vi "Filter Wheel GUI.vi"(9 "Standalone":bool=TRUE, 10 "Init Data":variant, 11 "Filter Wheel name":string="RIMAS") -> ()   [LabVIEW 2024]
uses:
  Filter Wheel Arduino Control/Filter Wheel Arduino Command cluster.ctl
  typedefs/CC enum Operation Mode.ctl
  Filter Wheel Arduino Control/Filter Wheel Arduino Homing cluster.ctl
  Filter Wheel Object/Filter Wheel.lvclass
  Filter Wheel configuration.ctl
  Filter Wheel Object/Filter Wheel Details.ctl
  Subsystems/SS typedef cluster Instrument Command Queue Data.ctl
  Subsystems/SS cluster Data Queue type.ctl
  FW cmd Q Move Parameters.ctl
  <vilib>/Utility/miscctls.llb/LVRowAndColumnTypeDef.ctl
  FW cluster Status.ctl
  FW enum status.ctl
  Filter Wheel Object/Filter Wheel.lvclass/Filter Wheel.ctl
  hk-channel-class/hk-channel-class/HK Item/HK Channel Units and Setup.ctl
  hk-channel-class/hk-channel-class/HK Item/HK Channel enum Data Type.ctl
  hk-channel-class/hk-channel-class/HK Item/HK Item.lvclass
  hk-channel-class/hk-channel-class/HK Item/HK Channel cluster Telemetry Data.ctl
  FW cmd Q Move Position Parameters.ctl
  typedefs/CC cluster Alarm Data.ctl
  Filter Wheel Arduino Control/FW Arduino Control.lvclass
  Filter Wheel Simulator/Filter Wheel Simulator.lvclass
  C:/Development/rimas/RIMAS/Filter Wheel/Filter Wheel Object/Filter Wheel.lvclass
  Filter Wheel Simulator/Filter Wheel Simulator.lvclass/Filter Wheel Simulator.ctl
panel:
  out "Messages":string
  in  "Mode":T1
  in  "Tab Control":T2(tab)
  out "Wheel Name":string
  out "Moving Message":string="Filter Wheel Moving...."
  in  "Error":bool
  out "Homed":bool[](array[boolean])
  in  "Wheel To Home":u16(ring) items=["FW YJ", "FW HK", "Aux", "Slit"]
  in  "STOP":bool
  out "Connected":bool
  in  "Filter Wheel Displays":T3 {"Gauge 0" scale=0.0..5.0; "Gauge 4" scale=0.0..5.0; "Gauge 3" scale=0.0..6.0; "Gauge 2" scale=0.0..5.0; "Gauge 5" scale=0.0..32768.0; "Gauge 8" scale=0.0..32768.0; "Gauge 6" scale=0.0..32768.0; "Gauge 7" scale=0.0..32768.0}
  in  "Home":bool
  out "Repeats":i32
  in  "Wheel ID":i32
  in  "Repeat Home":bool
  in  "Alarms?":bool=TRUE
  in  "Default Speed":u16=200 min=20 max=4000 step=10
  in  "Homing":T4[](array[typedef])
  in  "Sim Velocity (steps/sec)":i32
  in  "Connect":bool
  in  "Serial Port":refnum<visa-resource-name>="COM11"
  in  "Simulate":bool
  in  "Close":bool
  in  "Filter Wheel":u16(ring)
  in  "Slit Wheel Location":u16(ring)
  in  "Save Slit Wheel Pos":bool
  in  "Open Arduino Log":bool
  out "Moving":bool[](array[boolean])
  out "Last Move Positions":u32[](array[numeric])
  out "On the notch":bool[](array[boolean])
  in  "Filter Wheel Settings":T5={"Direction"=TRUE, "NUMBER OF  STEPS"=2900, "SPEED STEPS/SEC"=200, "ACC/DECEL STEPS/SEC^2"=400, "Move mode"=0, "EN/DIS?"=TRUE, "delay before \nread (ms)"=750, "Timeout before \nstop (ms)"=13000} {"Move mode" items=["Relative steps ##", "Search switch"]; "ACC/DECEL STEPS/SEC^2" max=4000; "SPEED STEPS/SEC" min=20 max=4000 step=10}
  in  "Command Preview":string
  out "Response":string
  in  "Send Command":bool
  in  "Read":bool
  in  "Restore Defaults":bool
  in  "Remove Pos":bool
  in  "Add Pos":bool
  in  "Save Button":bool
  in  "Remove Fw":bool
  in  "Add Fw":bool
  in  "Wheels":i32(listbox)
  in  "Positions":i32(listbox)
  # "Click for info"
  # "Home button will repeatedly home the wheel until it is pressed again. Repeats show number of homes done so far."
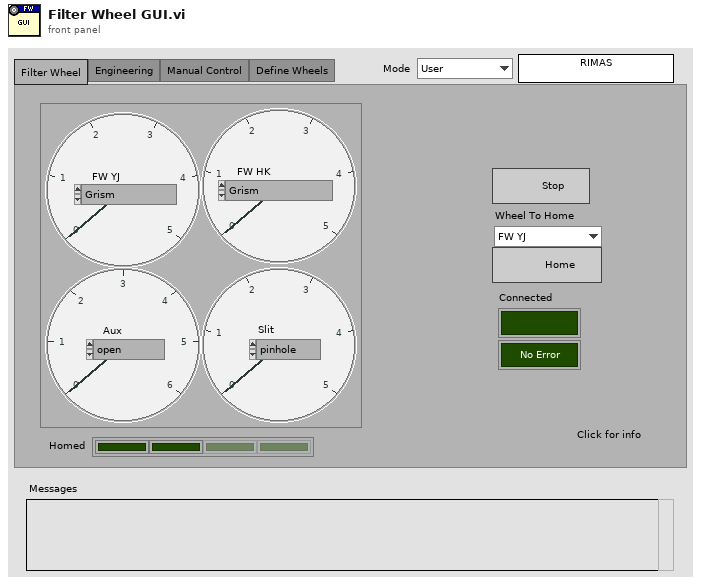
[diagram p1: front panel]
types:
  T1 = typedef "CC enum Operation Mode.ctl" = enum16{"User", "Engineering"}
  T2 = enum32{"Filter Wheel", "Engineering", "Manual Control", "Define Wheels"}
  T3 = cluster{"Gauge 0":i32, "Gauge 2":i32, "Gauge 3":i32, "Gauge 4":i32, "Gauge 5":i32, "Gauge 6":i32, "Gauge 7":i32, "Gauge 8":i32, "Position 0":i32, "Position 1":i32, "Position 2":i32, "Position 3":i32}
  T4 = typedef "Filter Wheel Arduino Homing cluster.ctl" = cluster{"Direction":bool, "Speed":i32, "Accel":i32, "Error Cnts":i32, "Homing Delta":i32}
  T5 = typedef "Filter Wheel Arduino Command cluster.ctl" = cluster{"Direction":bool, "NUMBER OF  STEPS":u32, "SPEED STEPS/SEC":u16, "ACC/DECEL STEPS/SEC^2":u16, "Move mode":u16, "EN/DIS?":bool, "delay before \nread (ms)":u32, "Timeout before \nstop (ms)":u32}
  T6 = typedef "SS typedef cluster Instrument Command Queue Data.ctl" = cluster{"Cmd":string, "Parameters":variant}
  T7 = typedef "Filter Wheel.lvclass/Filter Wheel configuration.ctl" = cluster{"Num Wheels":i32, "Filters":T8[], "Invalid Combinations":i32[][], "Addr":refnum<visa-resource-name>, "Name":string, "Simulate":bool, "Default Speed":u16, "Homing":T4[]}
  T8 = typedef "Filter Wheel.lvclass/Filter Wheel Details.ctl" = cluster{"Names":string[], "Relative Position":i32[], "Wheel Name":string, "Size":i32}
  T9 = typedef "FW cmd Q Move Parameters.ctl" = cluster{"Wheel ID":i32, "Position":i32}
  T10 = typedef "LVRowAndColumnTypeDef.ctl" = cluster{"Row":i32, "Column":i32}
  T11 = typedef "FW cluster Status.ctl" = cluster{"State":T12, "Positions":i32[], "Names":string[], "Notch":bool[], "Moving":bool[]}
  T12 = typedef "FW enum status.ctl" = enum16{"Initializing", "Moving", "Move Complete", "Error"}
  T13 = cluster{"state":refnum<user-event>, "Filter Wheel ref":refnum<class "Filter Wheel.lvclass">, "Filter Wheel Info":T7, "FW names":string[], "Pos Names":cluster{"Table":string[][]}[], "cmd q":refnum<queue>, "Cmd":T6, "Data Q":refnum<queue>, "Move":T9, "error":errorcluster, "next poll":timestamp, "FW refs":refnum<vi>[], "Wheel":i32, "Coords":T10, "fw name":string, "Simulate":bool, "ch names":string[][], "FW Status":T11, "Error State":string, "Name":string, "Period":dbl, "Home Repeats":i32}
  T14 = typedef "HK Item.lvclass/HK Channel Units and Setup.ctl" = cluster{"Unit Type":string, "Units":string, "Configuration":string, "Digits":i32, "Data Type":T15, "Exponential?":bool, "Source":string}
  T15 = typedef "HK Item.lvclass/HK Channel enum Data Type.ctl" = enum16{"Floating Point", "Integer", "Enum", "String", "Waveform", "File"}
  T16 = typedef "SS cluster Data Queue type.ctl" = cluster{"Source":string, "Type":string, "Data":variant}
  T17 = typedef "HK Item.lvclass/HK Channel cluster Telemetry Data.ctl" = cluster{"Ch Names":string[], "Ch Values":dbl[], "Timestamp":timestamp, "Data Type":T15}
  T18 = typedef "FW cmd Q Move Position Parameters.ctl" = cluster{"Position Names":string[]}
  T19 = enum32{"Page Enabled", "Page Disabled", "Page Disabled & Grayed"}
  T20 = typedef "CC cluster Alarm Data.ctl" = cluster{"Measured Value":dbl, "Alarm Low":dbl, "Alarm High":dbl, "Message":string, "Source":string}
  T21 = enum8{"Enabled", "Disabled", "Disabled and Grayed Out"}
  T22 = typedef "LVPoint32TypeDef.ctl" = cluster{"Horizontal":i32, "Vertical":i32}
  T23 = cluster{"Gauge 0":bool, "Gauge 2":bool, "Gauge 3":bool, "Gauge 4":bool, "Gauge 5":bool, "Gauge 6":bool, "Gauge 7":bool, "Gauge 8":bool, "Position 0":bool, "Position 1":bool, "Position 2":bool, "Position 3":bool}
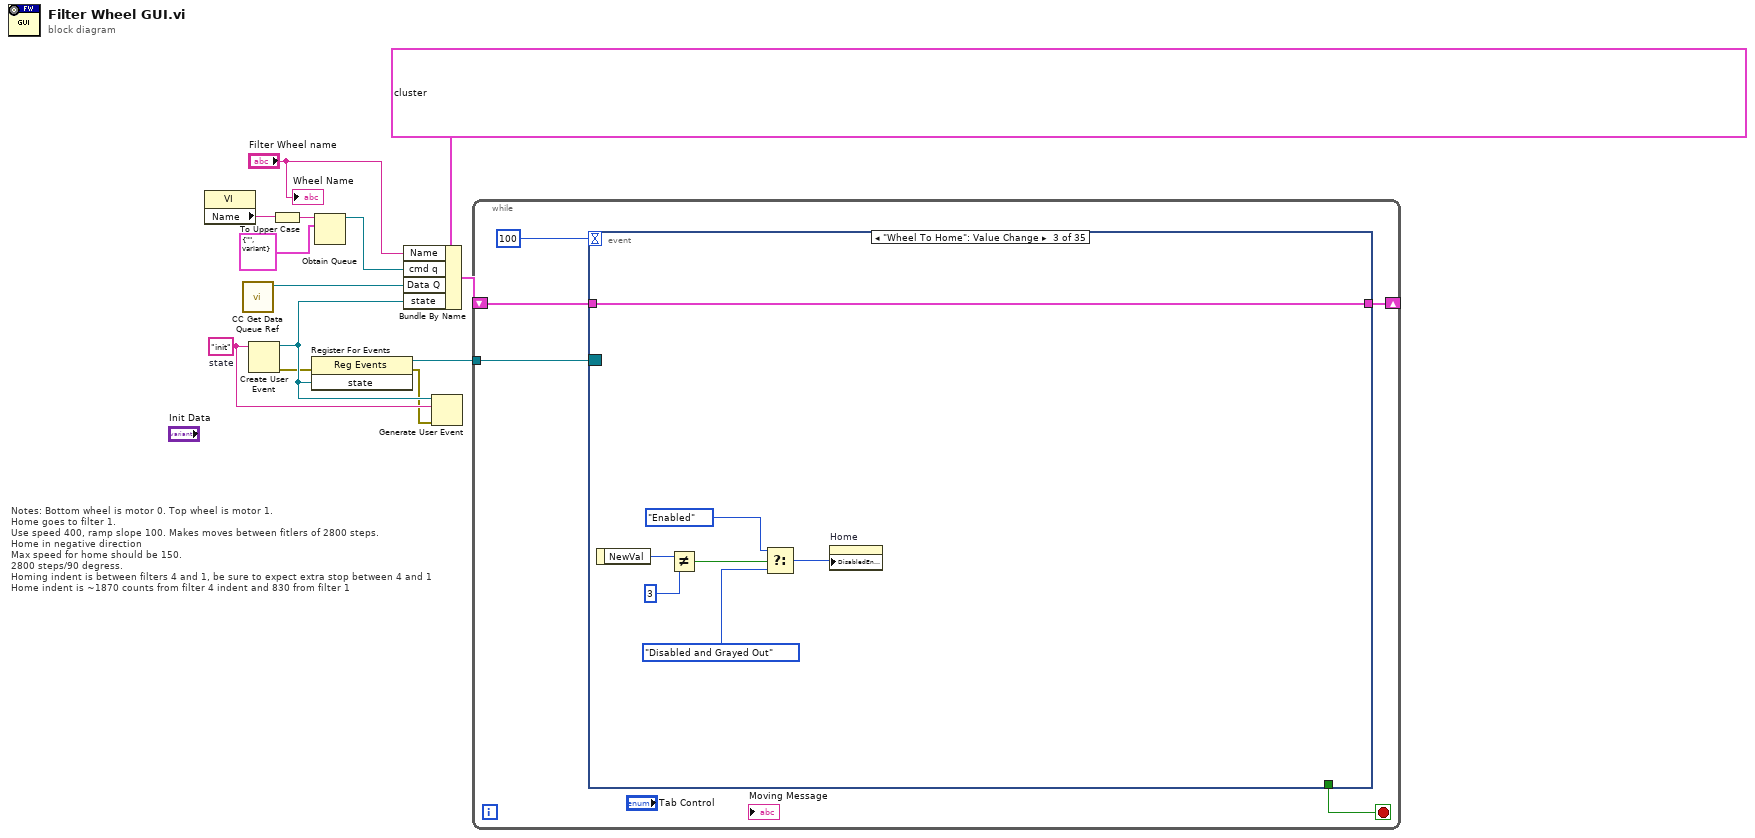
[diagram p0: block diagram]
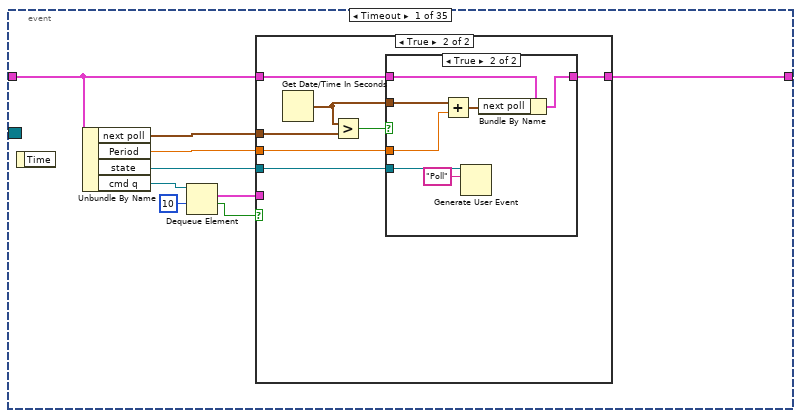
[diagram p2: hidden frame]
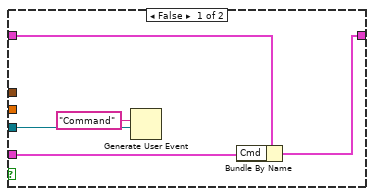
[diagram p3: hidden frame]
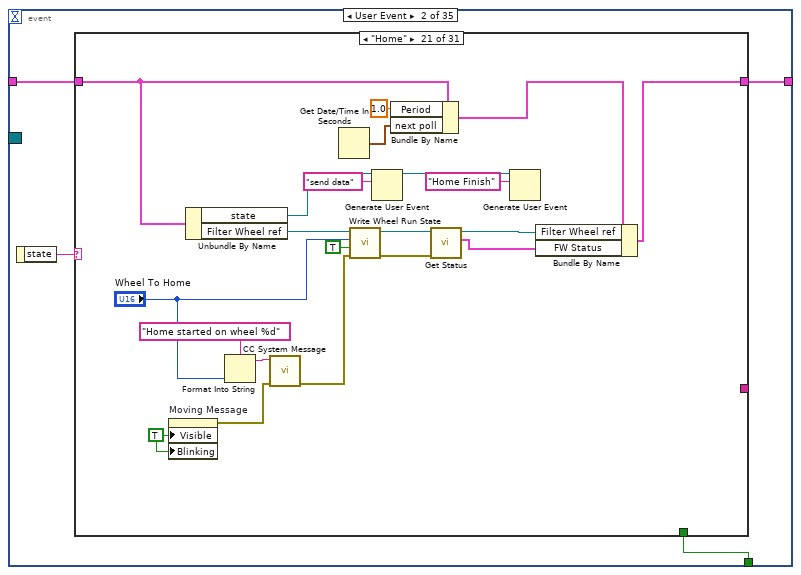
[diagram p5: hidden frame]
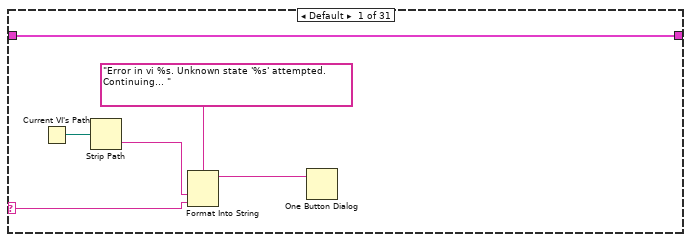
[diagram p6: hidden frame]
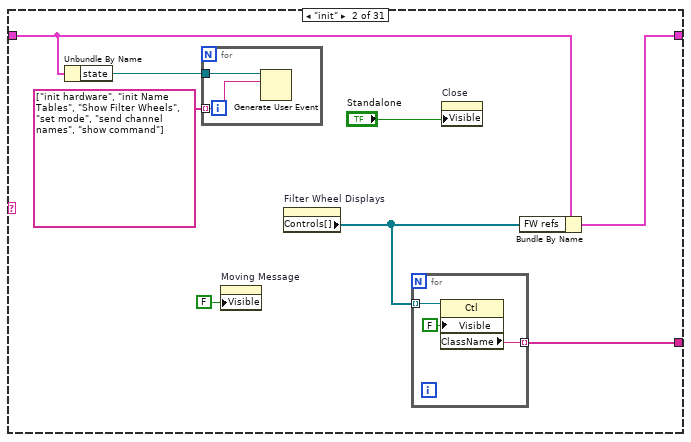
[diagram p7: hidden frame]
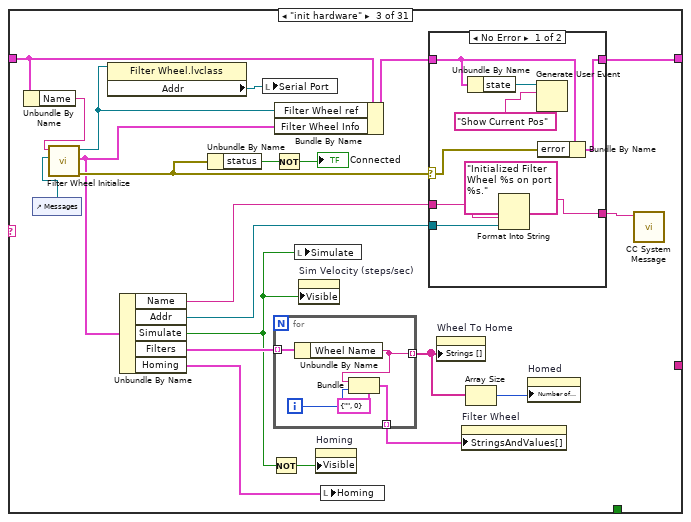
[diagram p8: hidden frame]
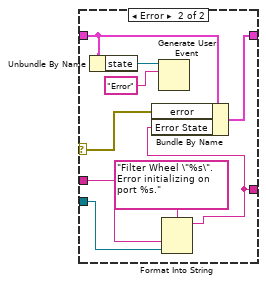
[diagram p9: hidden frame]
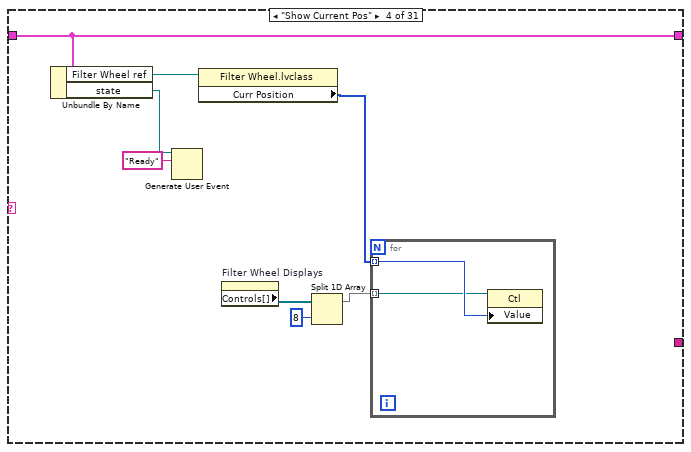
[diagram p10: hidden frame]
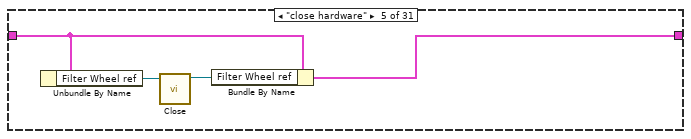
[diagram p11: hidden frame]
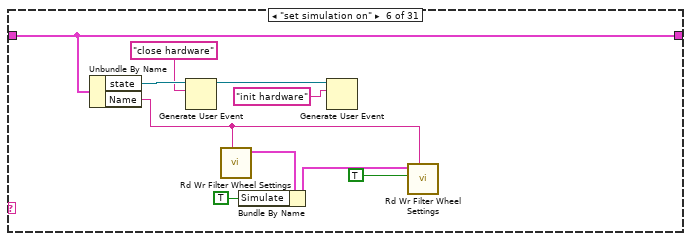
[diagram p12: hidden frame]
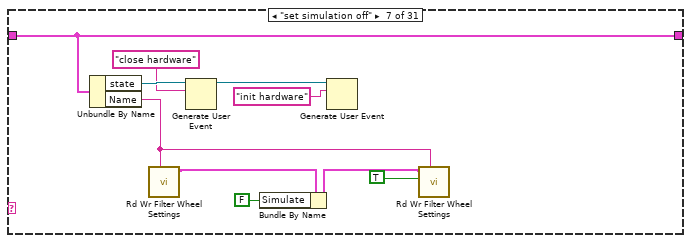
[diagram p13: hidden frame]
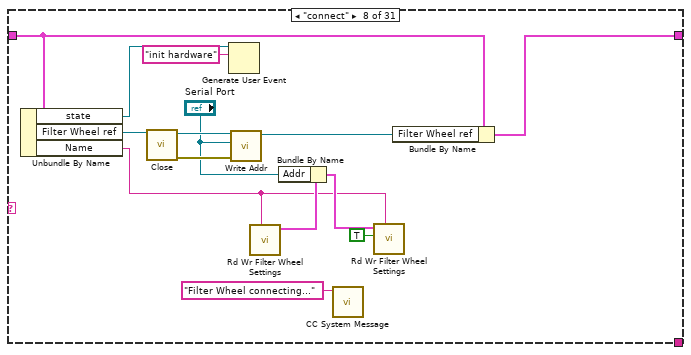
[diagram p14: hidden frame]
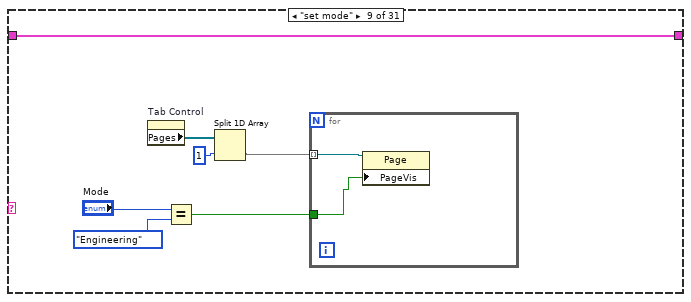
[diagram p15: hidden frame]
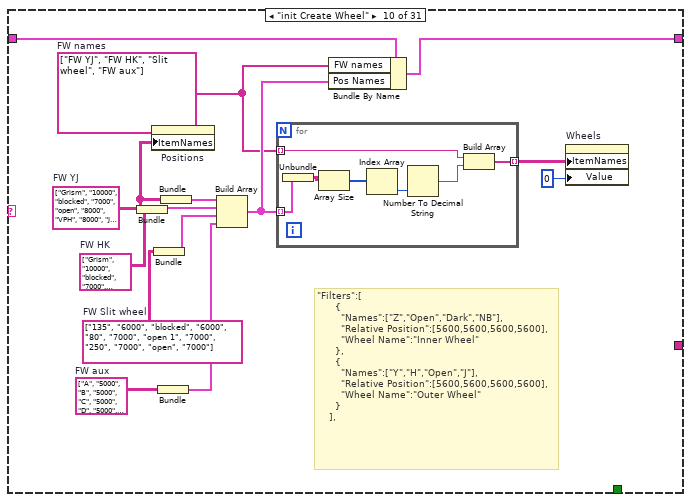
[diagram p16: hidden frame]
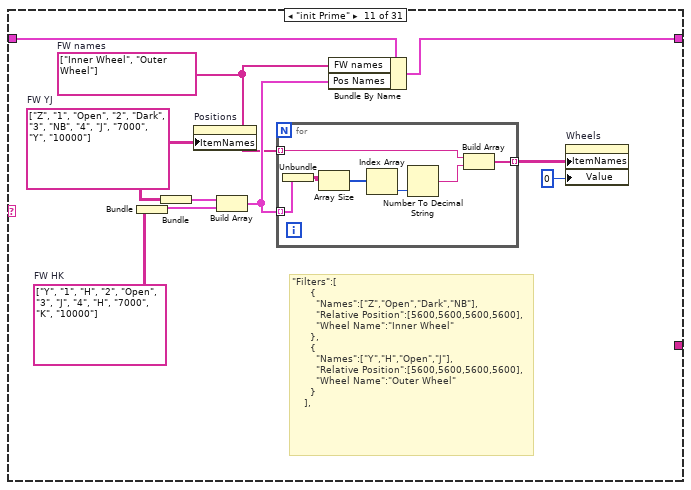
[diagram p17: hidden frame]
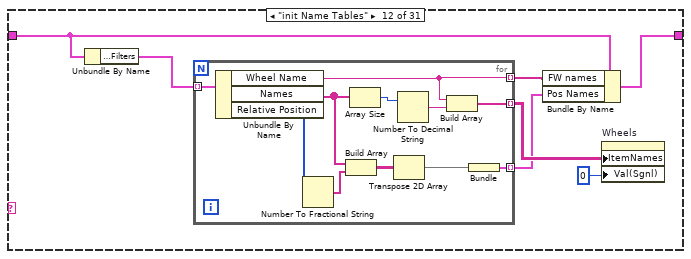
[diagram p18: hidden frame]
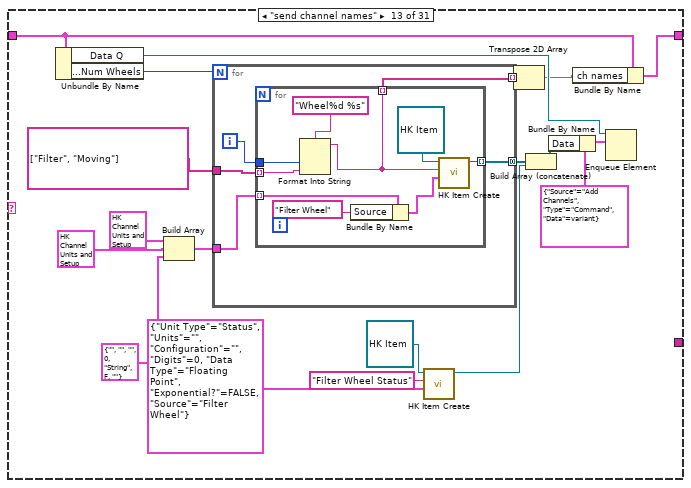
[diagram p19: hidden frame]
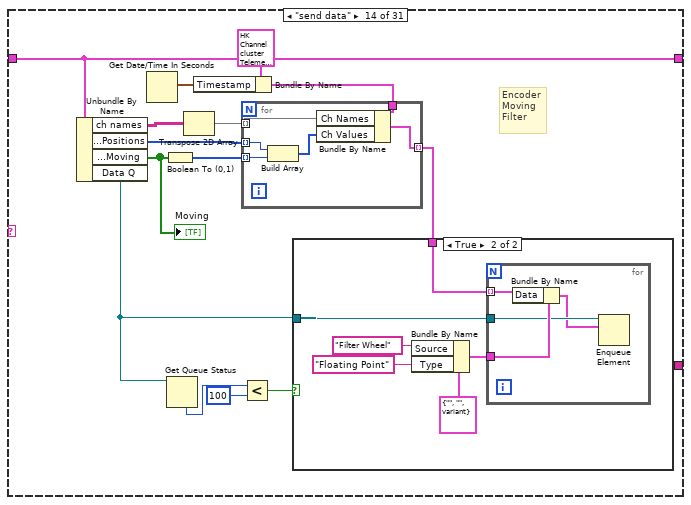
[diagram p20: hidden frame]
diagram:
  w9 = "init"  # state
  # "Notes: Bottom wheel is motor 0. Top wheel is motor 1.\nHome goes to filter 1. \nUse speed 400, ramp slope 100. Makes moves between fitlers of 2800 steps.\nHome in negative direction\nMax speed for home should be 150.\n2800 steps/90 degress.\nHoming indent is between filters 4 and 1, be sure to expect extra stop between 4 and 1\nHome indent is ~1870 counts from filter 4 indent and 830 from filter 1"
  n1 = property class="VI"() -> ("Name"=w5:string)  [unwired: 2 in, 2 out]
  n2 = call "CC Get Data Queue Ref.vi"() -> ("Data Q"=w6:refnum<queue>)  [unwired: 10 in, 1 out]
  n3 = Create User Event(user event datatype=w9) -> (user event=w11:refnum<user-event>, error out=w7:errorcluster)  [unwired: 1 in]
  n4 = To Upper Case(1:w5) -> (0:w4:string)
  n5 = register-events(error in=w7, w11) -> (reference out=w10:refnum<event-registration>, error out=w8:errorcluster)  [unwired: 1 in]
  n6 = Obtain Queue(name (unnamed)=w4, element data type=T6 {"Cmd"="", "Parameters"=variant}) -> (queue out=w2:refnum<queue>)  [unwired: 3 in, 2 out]
  n7 = Bundle By Name(cluster=T13 {"state"=refnum, "Filter Wheel ref"=refnum, "Filter Wheel Info"={"Num Wheels"=0, "Filters"=[], "Invalid Combinations"=[], "Addr"="", "Name"="", "Simulate"=FALSE, "Default Speed"=1000, "Homing"=[]}, "FW names"=["FW YJ", "FW HK", "Slit wheel", "FW aux"], "Pos Names"=[], "cmd q"=refnum, "Cmd"={"Cmd"="", "Parameters"=variant}, "Data Q"=refnum, "Move"={"Wheel ID"=0, "Position"=0}, "error"={"status"=FALSE, "code"=0, "source"=""}, "next poll"=timestamp(0 s since 1904-01-01), "FW refs"=[], "Wheel"=0, "Coords"={"Row"=0, "Column"=0}, "fw name"="", "Simulate"=TRUE, "ch names"=[], "FW Status"={"State"=enum."Move Complete", "Positions"=[], "Names"=[], "Notch"=[], "Moving"=[FALSE, FALSE]}, "Error State"="", "Name"="PRIME", "Period"=10.0, "Home Repeats"=0}, "Name"="Filter Wheel name", "cmd q"=w2, "Data Q"=w6, "state"=w11) -> (w12:T13)
  n8 = Generate User Event(user event=w11, event data cluster=w9, error in=w8) -> ()  [unwired: 1 in, 2 out]
  n9 = while {
    tunnel: w10 -> [w18]
    shift-right: [w17] -> _
    shift-left: w12 -> [w14]
    stop <- w16 stop-if-true
    n10 = event shown="[2] \"Wheel To Home\": Value Change" {
      selector: w18 -> [_ _ _ _ _ _ _ _ _ _ _ _ _ _ _ _ _ _ _ _ _ _ _ _ _ _ _ _ _ _ _ _ _ _ _]
      dyn-events: _ -> [_ _ _ _ _ _ _ _ _ _ _ _ _ _ _ _ _ _ _ _ _ _ _ _ _ _ _ _ _ _ _ _ _ _ _]
      timeout: 100 -> [_ _ _ _ _ _ _ _ _ _ _ _ _ _ _ _ _ _ _ _ _ _ _ _ _ _ _ _ _ _ _ _ _ _ _]
      tunnel: w14 -> [w22 w50 w608 w614 w618 w624 w644 w646 w655 w658 w660 w682 w689 w698 w701 w709 w710 w725 w728 w731 w734 w737 w746 w750 w757 w767 w789 w805 w827 w836 w842 w865 w878 w899 w903]
      tunnel: [w21 w49 w608 w613 w619 w625 w644 w645 w655 w658 w663 w683 w690 w698 w701 w709 w711 w725 w728 w731 w734 w737 w747 w751 w758 w768 w790 w806 w828 w837 w843 w866 w879 w899 w903] -> w17
      tunnel: [_ w48 _ _ _ _ _ _ _ _ _ _ _ _ _ _ _ _ _ _ _ _ _ _ _ _ _ _ _ _ _ _ _ _ _] -> w16
      event Timeout {
        n11 = event-data() -> ()  [unwired: 1 in, 1 out]
        n12 = Unbundle By Name(w22) -> ("next poll"=w20:timestamp, "Period"=w19:dbl, "state"=w23:refnum<user-event>, "cmd q"=w27:refnum<queue>)
        n13 = Dequeue Element(queue=w27, timeout in ms (-1)=10) -> (element=w24:T6, timed out?=w25:bool)  [unwired: 1 in, 2 out]
        n14 = case shown="True" w25 {
          tunnel: w24 -> [w29 _]
          tunnel: w23 -> [w32 w36]
          tunnel: w22 -> [w30 w37]
          tunnel: [w28 w34] -> w21
          tunnel: w20 -> [_ w39]
          tunnel: w19 -> [_ w33]
          frame False {
            n15 = Generate User Event(user event=w32, event data cluster="Command" ("event data")) -> ()  [unwired: 2 in, 2 out]
            n16 = Bundle By Name(cluster=w30, "Cmd"=w29) -> (w28:T13)
          }
          frame True {
            n17 = Get Date/Time In Seconds() -> (seconds since 1Jan1904=w35:timestamp)
            n18 = Greater?(x=w35, y=w39) -> (0:w38:bool)
            n19 = case shown="True" w38 {
              tunnel: w37 -> [w40 w47]
              tunnel: w36 -> [_ w46]
              tunnel: w35 -> [_ w45]
              tunnel: [w40 w43] -> w34
              tunnel: w33 -> [_ w41]
              frame False {
              }
              frame True {
                n20 = Add(x=w45, y=w41) -> (x+y=w44:timestamp)
                n21 = Generate User Event(user event=w46, event data cluster="Poll" ("event data")) -> ()  [unwired: 2 in, 2 out]
                n22 = Bundle By Name(cluster=w47, "next poll"=w44) -> (w43:T13)
              }
            }
          }
        }
      }
      event User Event {
        n23 = event-data() -> ("state"=w51:string)  [unwired: 1 in]
        n24 = case shown="\"Home\"" w51 {
          selector: w51 -> [w56 _ _ _ _ _ _ _ _ _ _ _ _ _ _ _ _ _ _ _ _ _ _ _ _ _ _ _ _ _ _]
          tunnel: w50 -> [w52 w64 w78 w122 w125 w137 w147 w158 w169 w172 w193 w214 w235 w274 w295 w308 w323 w332 w376 w442 w465 w494 w520 w533 w549 w557 w564 w571 w576 w597 w600]
          tunnel: [w52 w65 w90 w122 w126 w137 w147 w159 w169 w173 w194 w215 w236 w274 w295 w308 w323 w333 w383 w443 w483 w493 w521 w534 w550 w558 w564 w571 w577 w597 w600] -> w49
          tunnel: [_ _ _ _ _ _ _ _ _ _ _ _ _ _ _ _ _ _ _ _ _ _ _ _ _ _ _ _ _ _ TRUE] -> w48
          tunnel: [_ w58 _ _ _ _ _ _ _ _ _ _ _ _ _ _ _ _ _ _ _ _ _ _ _ _ _ _ _ _ _] -> _
          frame Default {
            n25 = Current VI's Path() -> (path=w55:path)
            n26 = Strip Path(path=w55) -> (name=w54:string)  [unwired: 1 out]
            n27 = Format Into String(format string="Error in vi %s. Unknown state '%s' attempted. Continuing... ", w54, w56) -> (resulting string=w53:string)  [unwired: 2 in, 1 out]
            n28 = One Button Dialog(message=w53) -> ()  [unwired: 1 in, 1 out]
          }
          frame "init" {
            n29 = Unbundle By Name(w64) -> ("state"=w63:refnum<user-event>)
            n30 = for {
              tunnel: w63 -> [w70]
              tunnel: string[] ["init hardware", "init Name Tables", "Show Filter Wheels", "set mode", "send channel names", "show command"] -> [w69] mode=indexing
              n31 = Generate User Event(user event=w70, event data cluster=w69) -> ()  [unwired: 2 in, 2 out]
            }
            n32 = property on="Moving Message" class="Str"("Visible"=FALSE) -> ()  [unwired: 2 in, 2 out]
            n33 = property on="Filter Wheel Displays" class="Clust (strict)"() -> ("Controls[]"=w60:refnum<vi>[])  [unwired: 2 in, 2 out]
            n34 = for {
              tunnel: w60 -> [w68] mode=indexing
              tunnel: [w66] -> w58 mode=indexing
              n35 = property class="Ctl"(reference=w68, "Visible"=FALSE) -> ("ClassName"=w66:string)  [unwired: 1 in, 2 out]
            }
            n36 = property on="Close" class="Bool"("Visible"="Standalone") -> ()  [unwired: 2 in, 2 out]
            n37 = Bundle By Name(cluster=w64, "FW refs"=w60) -> (w65:T13)
          }
          frame "init hardware" {
            n38 = Unbundle By Name(w78) -> ("Name"=w77:string)
            n39 = control-ref of="Messages"() -> (w72:refnum<vi>)
            n40 = call "Filter Wheel Initialize.vi"("Msg Ref"=w72, "Wheel Name"=w77) -> ("error out"=w89:errorcluster, "Filter Wheel Info"=w86:T7, "Filter Wheel.lvclass"=w74:refnum<class "Filter Wheel.lvclass">)  [unwired: 7 in]
            n41 = property class="Filter Wheel.lvclass"(reference=w74) -> ("Addr"=w73:refnum<visa-resource-name>)  [unwired: 1 in, 2 out]
            n42 = Unbundle By Name(w86) -> ("Name"=w85:string, "Addr"=w84:refnum<visa-resource-name>, "Simulate"=w75:bool, "Filters"=w82:T8[], "Homing"=w81:T4[])
            n43 = Unbundle By Name(w89) -> ("status"=w88:bool)
            n44 = local write "Serial Port"(w73) -> ()
            n45 = Not(x=w75) -> (.not. x?=w76:bool)
            n46 = Not(x=w88) -> (.not. x?=→"Connected":bool)
            n47 = for {
              tunnel: [w95] -> w80 mode=indexing
              tunnel: w82 -> [w96] mode=indexing
              tunnel: [w92] -> w71 mode=indexing
              i -> [w94]
              n48 = Unbundle By Name(w96) -> ("Wheel Name"=w95:string)
              n49 = Bundle(cluster=cluster{"String":string, "Value":u16} {"String"="", "Value"=0}, "String"=w95, "Value"=w94) -> (w92:cluster{"String":string, "Value":u16})
            }
            n50 = Bundle By Name(cluster=w78, "Filter Wheel ref"=w74, "Filter Wheel Info"=w86) -> (w91:T13)
            n51 = local write "Simulate"(w75) -> ()
            n52 = property on="Sim Velocity (steps/sec)" class="DigNum (strict)"("Visible"=w75) -> ()  [unwired: 2 in, 2 out]
            n53 = property on="Homing" class="Arr (strict)"("Visible"=w76) -> ()  [unwired: 2 in, 2 out]
            n54 = local write "Homing"(w81) -> ()
            n55 = case shown="No Error" w89 {
              selector: w89 -> [w99 w113]
              tunnel: [w98 w112] -> w90
              tunnel: w91 -> [w97 w111]
              tunnel: w85 -> [w104 w108]
              tunnel: w84 -> [w103 w107]
              tunnel: [w102 w106] -> w83
              frame No Error {
                n56 = Unbundle By Name(w97) -> ("state"=w100:refnum<user-event>)
                n57 = Format Into String(format string="Initialized Filter Wheel %s on port %s.", w104, w103) -> (resulting string=w102:string)  [unwired: 2 in, 1 out]
                n58 = Generate User Event(user event=w100, event data cluster="Show Current Pos" ("event data")) -> ()  [unwired: 2 in, 2 out]
                n59 = Bundle By Name(cluster=w97, "error"=w99) -> (w98:T13)
              }
              frame Error {
                n60 = Unbundle By Name(w111) -> ("state"=w110:refnum<user-event>)
                n61 = Generate User Event(user event=w110, event data cluster="Error" ("event data")) -> ()  [unwired: 2 in, 2 out]
                n62 = Format Into String(format string="Filter Wheel \"%s\". Error initializing on port %s.", w108, w107) -> (resulting string=w106:string)  [unwired: 2 in, 1 out]
                n63 = Bundle By Name(cluster=w111, "error"=w113, "Error State"=w106) -> (w112:T13)
              }
            }
            n64 = property on="Wheel To Home" class="Ring (strict)"("Strings []"=w80) -> ()  [unwired: 2 in, 2 out]
            n65 = property on="Filter Wheel" class="Ring (strict)"("StringsAndValues[]"=w71) -> ()  [unwired: 2 in, 2 out]
            n66 = Array Size(array=w80) -> (size(s)=w79:i32)
            n67 = property on="Homed" class="Arr (strict)"("Number of Columns"=w79) -> ()  [unwired: 2 in, 2 out]
            n68 = call "CC System Message.vi"("Message"=w83) -> ()  [unwired: 10 in, 1 out]
          }
          frame "Show Current Pos" {
            n69 = Unbundle By Name(w122) -> ("Filter Wheel ref"=w121:refnum<class "Filter Wheel.lvclass">, "state"=w120:refnum<user-event>)
            n70 = Generate User Event(user event=w120, event data cluster="Ready" ("event data")) -> ()  [unwired: 2 in, 2 out]
            n71 = property class="Filter Wheel.lvclass"(reference=w121) -> ("Curr Position"=w116:i32[])  [unwired: 1 in, 2 out]
            n72 = property on="Filter Wheel Displays" class="Clust (strict)"() -> ("Controls[]"=w118:refnum<vi>[])  [unwired: 2 in, 2 out]
            n73 = Split 1D Array(array=w118, index=8) -> (first subarray=w115:refnum<vi>[])  [unwired: 1 out]
            n74 = for {
              tunnel: w116 -> [w124] mode=indexing
              tunnel: w115 -> [w123] mode=indexing
              n75 = property class="Ctl"(reference=w123, "Value"=w124) -> ()  [unwired: 1 in, 2 out]
            }
          }
          frame "close hardware" {
            n76 = Unbundle By Name(w125) -> ("Filter Wheel ref"=w128:refnum<class "Filter Wheel.lvclass">)
            n77 = call-dynamic "Close.vi"("Filter Wheel in"=w128) -> ("Filter Wheel out"=w127:refnum<class "Filter Wheel.lvclass">)  [unwired: 9 in, 1 out]
            n78 = Bundle By Name(cluster=w125, "Filter Wheel ref"=w127) -> (w126:T13)
          }
          frame "set simulation on" {
            n79 = Unbundle By Name(w137) -> ("state"=w136:refnum<user-event>, "Name"=w129:string)
            n80 = Generate User Event(user event=w136, event data cluster="close hardware" ("event data")) -> (user event out=w135:refnum<user-event>)  [unwired: 2 in, 1 out]
            n81 = call "Rd Wr Filter Wheel Settings.vi"("Wheel Name"=w129) -> ("Filter Wheel Settings"=w132:T7)  [unwired: 9 in, 1 out]
            n82 = Bundle By Name(cluster=w132, "Simulate"=TRUE) -> (w131:T7)
            n83 = Generate User Event(user event=w135, event data cluster="init hardware" ("event data")) -> ()  [unwired: 2 in, 2 out]
            n84 = call "Rd Wr Filter Wheel Settings.vi"("Wheel Name"=w129, "Write? (F:Read)"=TRUE, "Filter Wheel Info"=w131) -> ()  [unwired: 7 in, 2 out]
          }
          frame "set simulation off" {
            n85 = Unbundle By Name(w147) -> ("state"=w146:refnum<user-event>, "Name"=w139:string)
            n86 = call "Rd Wr Filter Wheel Settings.vi"("Wheel Name"=w139) -> ("Filter Wheel Settings"=w142:T7)  [unwired: 9 in, 1 out]
            n87 = Generate User Event(user event=w146, event data cluster="close hardware" ("event data")) -> (user event out=w145:refnum<user-event>)  [unwired: 2 in, 1 out]
            n88 = Bundle By Name(cluster=w142, "Simulate"=FALSE) -> (w141:T7)
            n89 = Generate User Event(user event=w145, event data cluster="init hardware" ("event data")) -> ()  [unwired: 2 in, 2 out]
            n90 = call "Rd Wr Filter Wheel Settings.vi"("Wheel Name"=w139, "Write? (F:Read)"=TRUE, "Filter Wheel Info"=w141) -> ()  [unwired: 7 in, 2 out]
          }
          frame "connect" {
            n91 = Unbundle By Name(w158) -> ("state"=w156:refnum<user-event>, "Filter Wheel ref"=w162:refnum<class "Filter Wheel.lvclass">, "Name"=w149:string)
            n92 = call-dynamic "Close.vi"("Filter Wheel in"=w162) -> ("error out"=w160:errorcluster, "Filter Wheel out"=w161:refnum<class "Filter Wheel.lvclass">)  [unwired: 9 in]
            n93 = Generate User Event(user event=w156, event data cluster="init hardware" ("event data")) -> ()  [unwired: 2 in, 2 out]
            n94 = call "Write Addr.vi"("error in (no error)"=w160, "Addr"="Serial Port", "Filter Wheel in"=w161) -> ("Filter Wheel out"=w157:refnum<class "Filter Wheel.lvclass">)  [unwired: 7 in, 1 out]
            n95 = call "Rd Wr Filter Wheel Settings.vi"("Wheel Name"=w149) -> ("Filter Wheel Settings"=w154:T7)  [unwired: 9 in, 1 out]
            n96 = Bundle By Name(cluster=w154, "Addr"="Serial Port") -> (w152:T7)
            n97 = call "CC System Message.vi"("Message"="Filter Wheel connecting...") -> ()  [unwired: 10 in, 1 out]
            n98 = call "Rd Wr Filter Wheel Settings.vi"("Wheel Name"=w149, "Write? (F:Read)"=TRUE, "Filter Wheel Info"=w152) -> ()  [unwired: 7 in, 2 out]
            n99 = Bundle By Name(cluster=w158, "Filter Wheel ref"=w157) -> (w159:T13)
          }
          frame "set mode" {
            n100 = property on="Tab Control" class="TabCtl (strict)"() -> ("Pages"=w168:refnum<vi>[])  [unwired: 2 in, 2 out]
            n101 = Equal?(x="Mode", y=CC_enum_Operation_Mode."Engineering") -> (x = y?=w164:bool)
            n102 = Split 1D Array(array=w168, index=1) -> (second subarray=w163:refnum<vi>[])  [unwired: 1 out]
            n103 = for {
              tunnel: w163 -> [w171] mode=indexing
              tunnel: w164 -> [w170]
              n104 = property class="Page"(reference=w171, "PageVis"=w170) -> ()  [unwired: 1 in, 2 out]
            }
          }
          frame "init Create Wheel" {
            w174 = string[] ["FW YJ", "FW HK", "Slit wheel", "FW aux"]  # FW names
            w182 = string[][] [["Grism", "10000"], ["blocked", "7000"], ["open", "8000"], ["VPH", "8000"], ["J", "7000"], ["Y", "10000"]]  # FW YJ
            w185 = string[][] [["Grism", "10000"], ["blocked", "7000"], ["open", "8000"], ["VPH", "8000"], ["H", "7000"], ["K", "10000"]]  # FW HK
            w177 = string[][] [["135", "6000"], ["blocked", "6000"], ["80", "7000"], ["open 1", "7000"], ["250", "7000"], ["open", "7000"]]  # FW Slit wheel
            w184 = string[][] [["A", "5000"], ["B", "5000"], ["C", "5000"], ["D", "5000"], ["E", "5000"], ["F", "5000"], ["G", "5000"], ["H", "5000"]]  # FW aux
            # "\"Filters\":[\n      {\n        \"Names\":[\"Z\",\"Open\",\"Dark\",\"NB\"],\n        \"Relative Position\":[5600,5600,5600,5600],\n        \"Wheel Name\":\"Inner Wheel\"\n      },\n      {\n        \"Names\":[\"Y\",\"H\",\"Open\",\"J\"],\n        \"Relative Position\":[5600,5600,5600,5600],\n        \"Wheel Name\":\"Outer Wheel\"\n      }\n    ],"
            n105 = Bundle("FW HK"=w185) -> (w179:cluster{"FW HK":string[][]})  [unwired: 1 in]
            n106 = property on="Positions" class="MCListbox (strict)"("ItemNames"=w182) -> ()  [unwired: 2 in, 2 out]
            n107 = Bundle("FW Slit wheel"=w177) -> (w178:cluster{"FW Slit wheel":string[][]})  [unwired: 1 in]
            n108 = Bundle("FW aux"=w184) -> (w176:cluster{"FW aux":string[][]})  [unwired: 1 in]
            n109 = Bundle("FW YJ"=w182) -> (w180:cluster{"FW YJ":string[][]})  [unwired: 1 in]
            n110 = Build Array(w180, w179, w178, w176) -> (w175:cluster{"FW aux":string[][]}[])
            n111 = for {
              tunnel: w175 -> [w192] mode=indexing
              tunnel: w174 -> [w188] mode=indexing
              tunnel: [w187] -> w183 mode=indexing
              n112 = Unbundle(w192) -> ("FW aux"=w186:string[][])
              n113 = Array Size(array=w186) -> (size(s)=w191:i32[])
              n114 = Index Array(array=w191) -> (element=w190:i32)  [unwired: 1 in]
              n115 = Number To Decimal String(number=w190) -> (decimal integer string=w189:string)  [unwired: 1 in]
              n116 = Build Array(w188, w189) -> (w187:string[])
            }
            n117 = Bundle By Name(cluster=w172, "FW names"=w174, "Pos Names"=w175) -> (w173:T13)
            n118 = property on="Wheels" class="MCListbox (strict)"("ItemNames"=w183, "Value"=0 ("Wheels")) -> ()  [unwired: 2 in, 2 out]
          }
          frame "init Prime" {
            w195 = string[] ["Inner Wheel", "Outer Wheel"]  # FW names
            w200 = string[][] [["Z", "1"], ["Open", "2"], ["Dark", "3"], ["NB", "4"], ["J", "7000"], ["Y", "10000"]]  # FW YJ
            w202 = string[][] [["Y", "1"], ["H", "2"], ["Open", "3"], ["J", "4"], ["H", "7000"], ["K", "10000"]]  # FW HK
            # "\"Filters\":[\n      {\n        \"Names\":[\"Z\",\"Open\",\"Dark\",\"NB\"],\n        \"Relative Position\":[5600,5600,5600,5600],\n        \"Wheel Name\":\"Inner Wheel\"\n      },\n      {\n        \"Names\":[\"Y\",\"H\",\"Open\",\"J\"],\n        \"Relative Position\":[5600,5600,5600,5600],\n        \"Wheel Name\":\"Outer Wheel\"\n      }\n    ],"
            n119 = Bundle("FW HK"=w202) -> (w197:cluster{"FW HK":string[][]})  [unwired: 1 in]
            n120 = Bundle("FW YJ"=w200) -> (w198:cluster{"FW YJ":string[][]})  [unwired: 1 in]
            n121 = property on="Positions" class="MCListbox (strict)"("ItemNames"=w200) -> ()  [unwired: 2 in, 2 out]
            n122 = Build Array(w198, w197) -> (w196:cluster{"FW HK":string[][]}[])
            n123 = for {
              tunnel: w196 -> [w209] mode=indexing
              tunnel: w195 -> [w205] mode=indexing
              tunnel: [w204] -> w201 mode=indexing
              n124 = Unbundle(w209) -> ("FW HK"=w203:string[][])
              n125 = Array Size(array=w203) -> (size(s)=w208:i32[])
              n126 = Index Array(array=w208) -> (element=w207:i32)  [unwired: 1 in]
              n127 = Number To Decimal String(number=w207) -> (decimal integer string=w206:string)  [unwired: 1 in]
              n128 = Build Array(w205, w206) -> (w204:string[])
            }
            n129 = Bundle By Name(cluster=w193, "FW names"=w195, "Pos Names"=w196) -> (w194:T13)
            n130 = property on="Wheels" class="MCListbox (strict)"("ItemNames"=w201, "Value"=0 ("Wheels")) -> ()  [unwired: 2 in, 2 out]
          }
          frame "init Name Tables" {
            n131 = Unbundle By Name(w214) -> ("Filter Wheel Info.Filters"=w213:T8[])
            n132 = for {
              tunnel: w213 -> [w227] mode=indexing
              tunnel: [w224] -> w212 mode=indexing
              tunnel: [w223] -> w211 mode=indexing
              tunnel: [w218] -> w210 mode=indexing
              n133 = Unbundle By Name(w227) -> ("Wheel Name"=w224:string, "Names"=w220:string[], "Relative Position"=w222:i32[])
              n134 = Number To Fractional String(number=w222) -> (F-format string=w221:string[])  [unwired: 3 in]
              n135 = Build Array(w220, w221) -> (w219:string[][])
              n136 = Array Size(array=w220) -> (size(s)=w226:i32)
              n137 = Transpose 2D Array(2D array=w219) -> (transposed array=w217:string[][])
              n138 = Number To Decimal String(number=w226) -> (decimal integer string=w225:string)  [unwired: 1 in]
              n139 = Build Array(w224, w225) -> (w223:string[])
              n140 = Bundle(w217) -> (w218:cluster{string[][]})  [unwired: 1 in]
            }
            n141 = Bundle By Name(cluster=w214, "FW names"=w212, "Pos Names"=w210) -> (w215:T13)
            n142 = property on="Wheels" class="MCListbox (strict)"("ItemNames"=w211, "Val(Sgnl)"=0 ("Wheels")) -> ()  [unwired: 2 in, 2 out]
          }
          frame "send channel names" {
            n143 = Unbundle By Name(w235) -> ("Data Q"=w239:refnum<queue>, "Filter Wheel Info.Num Wheels"=w238:i32)
            n144 = Build Array(T14 {"Unit Type"="", "Units"="Counts", "Configuration"="", "Digits"=0, "Data Type"=enum."Integer", "Exponential?"=FALSE, "Source"=""} ("Channel Setup"), T14 {"Unit Type"="", "Units"="OnOff", "Configuration"="", "Digits"=0, "Data Type"=enum."Integer", "Exponential?"=FALSE, "Source"=""} ("Channel Setup"), T14 {"Unit Type"="", "Units"="", "Configuration"="", "Digits"=0, "Data Type"=enum."String", "Exponential?"=FALSE, "Source"=""} ("Channel Setup")) -> (w242:T14[])
            n145 = for {
              N: w238 -> [_]
              tunnel: string[] ["Filter", "Moving"] -> [w251]
              tunnel: w242 -> [w250]
              tunnel: [w249] -> w237 mode=concatenating
              tunnel: [w247] -> w234 mode=indexing
              i -> [w248]
              n146 = for {
                tunnel: w251 -> [w258] mode=indexing
                tunnel: w250 -> [w253] mode=indexing
                tunnel: [w257] -> w249 mode=indexing
                tunnel: w248 -> [w256]
                tunnel: [w255] -> w247 mode=indexing
                n147 = Format Into String(format string="Wheel%d %s", w256, w258) -> (resulting string=w255:string)  [unwired: 2 in, 1 out]
                n148 = Bundle By Name(cluster=w253, "Source"="Filter Wheel") -> (w254:T14)
                n149 = call-dynamic "HK Item Create.vi"("Channel Setup"=w254, "Name"=w255, "HK Item in"=refnum<class "HK Item.lvclass"> refnum) -> ("HK Item out"=w257:refnum<class "HK Item.lvclass">)  [unwired: 7 in, 1 out]
              }
            }
            n150 = call-dynamic "HK Item Create.vi"("Channel Setup"=T14 {"Unit Type"="Status", "Units"="", "Configuration"="", "Digits"=0, "Data Type"=enum."Floating Point", "Exponential?"=FALSE, "Source"="Filter Wheel"}, "Name"="Filter Wheel Status", "HK Item in"=refnum<class "HK Item.lvclass"> refnum) -> ("HK Item out"=w228:refnum<class "HK Item.lvclass">)  [unwired: 7 in, 1 out]
            n151 = Transpose 2D Array(2D array=w234) -> (transposed array=w233:string[][])
            n152 = Build Array (concatenate)(w237, w228) -> (w229:refnum<class "HK Item.lvclass">[])
            n153 = Bundle By Name(cluster=T16 {"Source"="Add Channels", "Type"="Command", "Data"=variant} ("element"), "Data"=w229) -> (w241:T16)
            n154 = Bundle By Name(cluster=w235, "ch names"=w233) -> (w236:T13)
            n155 = Enqueue Element(queue=w239, element=w241) -> ()  [unwired: 2 in, 3 out]
          }
          frame "send data" {
            # "Encoder\nMoving\nFilter"
            n156 = Unbundle By Name(w274) -> ("ch names"=w268:string[][], "FW Status.Positions"=w263:i32[], "FW Status.Moving"=w269:bool[], "Data Q"=w272:refnum<queue>)
            "Moving" <- w269
            n157 = Get Date/Time In Seconds() -> (seconds since 1Jan1904=w266:timestamp)
            n158 = Boolean To (0,1)(Boolean=w269) -> (0, 1=w264:i16[])
            n159 = Get Queue Status(queue=w272) -> (# elements in queue=w271:i32)  [unwired: 2 in, 7 out]
            n160 = Transpose 2D Array(2D array=w268) -> (transposed array=w261:string[][])
            n161 = Bundle By Name(cluster=T17 {"Ch Names"=[], "Ch Values"=[], "Timestamp"=timestamp(0 s since 1904-01-01), "Data Type"=enum."Integer"}, "Timestamp"=w266) -> (w265:T17)
            n162 = for {
              tunnel: [w280] -> w273 mode=indexing
              tunnel: w261 -> [w279] mode=indexing
              tunnel: w265 -> [w278]
              tunnel: w264 -> [w277] mode=indexing
              tunnel: w263 -> [w276] mode=indexing
              n163 = Build Array(w276, w277) -> (w275:i32[])
              n164 = Bundle By Name(cluster=w278, "Ch Names"=w279, "Ch Values"=w275) -> (w280:T17)
            }
            n165 = Less?(x=w271, y=100) -> (x < y?=w262:bool)
            n166 = case shown="True" w262 {
              tunnel: w273 -> [_ w282]
              tunnel: w272 -> [_ w281]
              frame False {
              }
              frame True {
                n167 = Bundle By Name(cluster=T16 {"Source"="", "Type"="", "Data"=variant} ("element"), "Source"="Filter Wheel", "Type"="Floating Point" ("Data Type")) -> (w283:T16)
                n168 = for {
                  tunnel: w283 -> [w290]
                  tunnel: w282 -> [w289] mode=indexing
                  tunnel: w281 -> [w288]
                  n169 = Bundle By Name(cluster=w290, "Data"=w289) -> (w287:T16)
                  n170 = Enqueue Element(queue=w288, element=w287) -> ()  [unwired: 2 in, 3 out]
                }
              }
            }
          }
          frame "Show Tables" {
            n171 = Unbundle By Name(w295) -> ("FW names"=w294:string[], "Pos Names"=w293:cluster{"Table":string[][]}[])
            n172 = for {
              tunnel: w294 -> [w297] mode=indexing
              tunnel: w293 -> [w301] mode=indexing
              tunnel: [w296] -> w291 mode=indexing
              n173 = Unbundle By Name(w301) -> ("Table"=w300:string[][])
              n174 = Array Size(array=w300) -> (size(s)=w299:i32[])
              n175 = Number To Decimal String(number=w299) -> (decimal integer string=w298:string[])  [unwired: 1 in]
              n176 = Build Array (concatenate)(w297, w298) -> (w296:string[])
            }
            n177 = property on="Wheels" class="MCListbox (strict)"("ItemNames"=w291, "Val(Sgnl)"=0 ("Wheels")) -> ()  [unwired: 2 in, 2 out]
          }
          frame "Show Filter Wheels" {
            (unwired) string[] ["Grism", "blocked", "VPH", "open", "J", "Y"] ("Array")
            n178 = Unbundle By Name(w308) -> ("Filter Wheel Info.Filters"=w305:T8[], "FW refs"=w307:refnum<vi>[])
            n179 = Index Array(array=w305, index=3) -> (element=w304:T8)
            n180 = for {
              tunnel: w305 -> [w321] mode=indexing
              tunnel: w307 -> [w320] mode=indexing
              tunnel: [w315] -> w306 mode=indexing
              w311 = TRUE ("Visible")
              n181 = Unbundle By Name(w321) -> ("Wheel Name"=w317:string, "Names"=w312:string[], "Size"=w310:i32)
              n182 = control-ref of="Gauge 0"() -> (w318:refnum<vi>)
              n183 = To More Specific Class(target class=w318, reference=w320) -> (specific class reference=w319:refnum<vi>)  [unwired: 1 in, 1 out]
              n184 = property class="Knob (strict)"(reference=w319, "Visible"=w311, "TextLbls[]"=w312, "Caption.Text"=w317, "Visible"=w311) -> (error out=w313:errorcluster)  [unwired: 1 in, 1 out]
              n185 = Array Size(array=w312) -> (size(s)=w316:i32)
              n186 = Number To Decimal String(number=w316) -> (decimal integer string=w314:string)  [unwired: 1 in]
              n187 = Number To Decimal String(number=w310) -> (decimal integer string=w309:string)  [unwired: 1 in]
              n188 = Build Array(w317, w314, w309) -> (w315:string[])
              n189 = call <vilib>:"Clear Errors.vi"("error in (no error)"=w313) -> ()  [unwired: 5 in, 2 out]
            }
            n190 = Unbundle By Name(w304) -> ("Names"=w303:string[])
            n191 = property on="Slit Wheel Location" class="Ring (strict)"("Strings []"=w303) -> ()  [unwired: 2 in, 2 out]
            n192 = property on="Wheels" class="MCListbox (strict)"("ItemNames"=w306) -> ()  [unwired: 2 in, 2 out]
          }
          frame "show command" {
            n193 = call "Arduino Generate Command String.vi"("Filter Wheel Settings"="Filter Wheel Settings", "MOTOR NUMBER"="Filter Wheel") -> ("Cmd String"=w325:string)  [unwired: 9 in]
            n194 = property on="Command Preview" class="Str"("Value"=w325) -> ()  [unwired: 2 in, 2 out]
          }
          frame "Command" {
            n195 = Unbundle By Name(w332) -> ("state"=w334:refnum<user-event>, "Data Q"=w335:refnum<queue>, "Cmd.Cmd"=w330:string, "Cmd.Parameters"=w328:variant)
            n196 = Variant To Flattened String(Variant=w328) -> (data string=w329:string)  [unwired: 1 out]
            n197 = Format Into String(format string="Filter Wheel Command %s. Parameters %s" ("Message"), w330, w329) -> (resulting string=w327:string)  [unwired: 2 in, 1 out]
            n198 = call "CC System Message.vi"("Message"=w327) -> ("error out"=w326:errorcluster)  [unwired: 10 in]
            n199 = case shown="\"Move\"" w330 {
              selector: w330 -> [w345 _ _ _ _ _]
              tunnel: w335 -> [w350 _ _ _ _ _]
              tunnel: w328 -> [_ w360 w364 _ _ _]
              tunnel: w334 -> [w339 w356 _ w367 w369 w373]
              tunnel: w332 -> [w343 w351 w361 w365 w368 w371]
              tunnel: [w337 w357 w361 w365 w368 w371] -> w333
              tunnel: w326 -> [_ _ _ _ _ _]
              frame "False", Default {
                n200 = Generate User Event(user event=w339, event data cluster="Error" ("event data")) -> ()  [unwired: 2 in, 2 out]
                n201 = Format Into String(format string="Filter Wheel received invalid command. Cmd: %s", w345) -> (resulting string=w342:string)  [unwired: 2 in, 1 out]
                n202 = call "lib Quick Message Log.vi"("Message"=w345) -> ("Log"=→"Messages":string)  [unwired: 9 in, 1 out]
                n203 = Bundle By Name(cluster=T16 {"Source"="", "Type"="", "Data"=variant} ("element"), "Source"="Message" ("Data Type"), "Data"=w342) -> (w346:T16)
                n204 = Bundle By Name(cluster=w343, "Error State"="Command", "error.status"=TRUE, "error.code"=5000, "error.source"=w342) -> (w337:T13)
                n205 = Enqueue Element(queue=w350, element=w346) -> ()  [unwired: 2 in, 3 out]
              }
              frame "Move" {
                n206 = Generate User Event(user event=w356, event data cluster="Move" ("event data")) -> ()  [unwired: 2 in, 2 out]
                n207 = Get Date/Time In Seconds() -> (seconds since 1Jan1904=w353:timestamp)
                n208 = Bundle By Name(cluster=w351, "Period"=1.0, "next poll"=w353) -> (w352:T13)
                n209 = Variant To Data(type=T9 {"Wheel ID"=0, "Position"=0}, Variant=w360) -> (data=w358:T9)  [unwired: 1 in, 1 out]
                n210 = Bundle By Name(cluster=w352, "Move"=w358) -> (w357:T13)
              }
              frame "MoveFilter" {
                n211 = Variant To Data(type=T18 {"Position Names"=[]}, Variant=w364) -> (data=w362:T18)  [unwired: 1 in, 1 out]
                n212 = Unbundle By Name(w362) -> ()  [unwired: 1 out]
              }
              frame "Status" {
                n213 = Generate User Event(user event=w367, event data cluster="Send Status" ("event data")) -> ()  [unwired: 2 in, 2 out]
              }
              frame "Config" {
                n214 = Generate User Event(user event=w369, event data cluster="Send Config" ("event data")) -> ()  [unwired: 2 in, 2 out]
              }
              frame "Shutdown" {
                n215 = Generate User Event(user event=w373, event data cluster="Shutdown" ("event data")) -> ()  [unwired: 2 in, 2 out]
              }
            }
          }
          frame "Move" {
            n216 = Unbundle By Name(w376) -> ("state"=w384:refnum<user-event>, "Filter Wheel ref"=w375:refnum<class "Filter Wheel.lvclass">, "Move"=w386:T9, "Filter Wheel Info"=w385:T7)
            n217 = Get Date/Time In Seconds() -> (seconds since 1Jan1904=w378:timestamp)
            n218 = call "Filter Wheel Validate Move Command.vi"("Filter Wheel in"=w375, "Filter Wheel Info"=w385, "Move"=w386) -> ("error out"=w381:errorcluster, "already in pos?"=w374:bool, "Move dup"=w380:T9)  [unwired: 5 in, 1 out]
            n219 = Bundle By Name(cluster=w376, "Period"=1.0, "next poll"=w378) -> (w377:T13)
            n220 = case shown="No Error" w381 {
              selector: w381 -> [_ w418]
              tunnel: w384 -> [w393 w424]
              tunnel: w377 -> [w389 w422]
              tunnel: [w390 w421] -> w383
              tunnel: [w388 w419] -> w382
              tunnel: w375 -> [w392 _]
              tunnel: w380 -> [w391 _]
              tunnel: w374 -> [w387 _]
              frame No Error {
                n221 = case shown="False" w387 {
                  tunnel: w393 -> [w414 _]
                  tunnel: w392 -> [w413 _]
                  tunnel: w391 -> [w412 _]
                  tunnel: [w410 w416] -> w390
                  tunnel: w389 -> [w409 w416]
                  tunnel: [w400 "Filter wheel already in position."] -> w388
                  frame False {
                    w398 = TRUE ("Visible")
                    n222 = Unbundle By Name(w412) -> ("Wheel ID"=w402:i32, "Position"=w401:i32)
                    n223 = property on="Tab Control" class="TabCtl (strict)"() -> ("Pages"=w397:refnum<vi>[])  [unwired: 2 in, 2 out]
                    n224 = Index Array(array=w397, index=0) -> (element=w396:refnum<vi>)
                    n225 = call-dynamic "Write Wheel Run State.vi"("Run"=TRUE, "Wheel"=w402, "Filter Wheel in"=w413) -> ("Filter Wheel out"=w405:refnum<class "Filter Wheel.lvclass">)  [unwired: 7 in, 1 out]
                    n226 = Generate User Event(user event=w414, event data cluster="send data" ("event data")) -> (user event out=w407:refnum<user-event>)  [unwired: 2 in, 1 out]
                    n227 = call-dynamic "Get Status.vi"("Filter Wheel in"=w405) -> ("FW Status"=w399:T11, "Filter Wheel out"=w404:refnum<class "Filter Wheel.lvclass">)  [unwired: 8 in, 1 out]
                    n228 = property class="Page"(reference=w396, "PageEnb"=T19."Page Disabled & Grayed" ("Page Enabled State")) -> ()  [unwired: 1 in, 2 out]
                    n229 = Format Into String(format string="Initiating filter wheel %d move to position %d.", w402, w401) -> (resulting string=w400:string)  [unwired: 2 in, 1 out]
                    n230 = Generate User Event(user event=w407, event data cluster="Move Finish" ("event data")) -> ()  [unwired: 2 in, 2 out]
                    n231 = Bundle By Name(cluster=w409, "Filter Wheel ref"=w404, "FW Status"=w399) -> (w410:T13)
                    n232 = property on="Moving Message" class="Str"("Visible"=w398, "Blinking"=w398) -> ()  [unwired: 2 in, 2 out]
                  }
                  frame True {
                  }
                }
              }
              frame Error {
                n233 = Generate User Event(user event=w424, event data cluster="Error" ("event data")) -> ()  [unwired: 2 in, 2 out]
                n234 = Unbundle By Name(w418) -> ("source"=w417:string)
                n235 = Format Into String(format string="Filter Wheel Move Error: %s", w417) -> (resulting string=w419:string)  [unwired: 2 in, 1 out]
                n236 = Bundle By Name(cluster=w422, "error"=w418, "Error State"=w419) -> (w421:T13)
              }
            }
            n237 = call "CC System Message.vi"("Message"=w382) -> ()  [unwired: 10 in, 1 out]
          }
          frame "Move Finish" {
            w437 = FALSE ("Visible")
            n238 = Unbundle By Name(w442) -> ("state"=w444:refnum<user-event>, "Filter Wheel ref"=w447:refnum<class "Filter Wheel.lvclass">, "Move"=w436:T9)
            n239 = property on="Tab Control" class="TabCtl (strict)"() -> ("Pages"=w435:refnum<vi>[])  [unwired: 2 in, 2 out]
            n240 = local read "Last Move Positions"() -> (w428:u32[])
            n241 = Unbundle By Name(w436) -> ("Wheel ID"=w426:i32, "Position"=w445:i32)
            n242 = Index Array(array=w435, index=0) -> (element=w433:refnum<vi>)
            n243 = call-dynamic "Set One Filter.vi"("Position (0:4)"=w445, "Filter Wheel (0:n-1)"=w426, "Filter Wheel in"=w447) -> ("error out"=w429:errorcluster, "Target Counts"=w425:i32, "Filter Wheel out"=w432:refnum<class "Filter Wheel.lvclass">, "Message"=w440:string)  [unwired: 3 in, 2 out]
            n244 = Replace Array Subset(array=w428, new element=w425, index=w426) -> (→"Last Move Positions":u32[])
            n245 = call-dynamic "Write Wheel Run State.vi"("Run"=FALSE, "Wheel"=w426, "Filter Wheel in"=w432) -> ("Filter Wheel out"=w430:refnum<class "Filter Wheel.lvclass">)  [unwired: 7 in, 1 out]
            n246 = case shown="No Error" w429 {
              selector: w429 -> [_ w461]
              tunnel: w444 -> [_ w464]
              tunnel: w442 -> [w453 w462]
              tunnel: [w451 w460] -> w443
              tunnel: w433 -> [w454 w459]
              tunnel: [w454 w459] -> w441
              tunnel: w430 -> [w452 w455]
              tunnel: w440 -> [w449 w457]
              tunnel: ["Move complete." ("string") w456] -> w439
              frame No Error {
                n247 = call "CC System Message.vi"("Message"=w449) -> ()  [unwired: 10 in, 1 out]
                n248 = Bundle By Name(cluster=w453, "Filter Wheel ref"=w452, "Period"=30.0) -> (w451:T13)
              }
              frame Error {
                n249 = Generate User Event(user event=w464, event data cluster="Error" ("event data")) -> ()  [unwired: 2 in, 2 out]
                n250 = Format Into String(format string="Filter Wheel Move Error: %s", w457) -> (resulting string=w456:string)  [unwired: 2 in, 1 out]
                n251 = Bundle By Name(cluster=w462, "Filter Wheel ref"=w455, "error"=w461, "Error State"=w456) -> (w460:T13)
              }
            }
            n252 = property class="Page"(reference=w441, "PageEnb"=T19."Page Enabled" ("Page Enabled State")) -> (error out=w438:errorcluster)  [unwired: 1 in, 1 out]
            n253 = property on="Moving Message" class="Str"(error in=w438, "Visible"=w437, "Blinking"=w437) -> ()  [unwired: 1 in, 2 out]
            n254 = call "CC System Message.vi"("Message"=w439) -> ()  [unwired: 10 in, 1 out]
          }
          frame "Home" {
            w482 = TRUE ("Visible")
            n255 = property on="Moving Message" class="Str"("Visible"=w482, "Blinking"=w482) -> (error out=w481:errorcluster)  [unwired: 2 in, 1 out]
            n256 = Unbundle By Name(w465) -> ("state"=w476:refnum<user-event>, "Filter Wheel ref"=w480:refnum<class "Filter Wheel.lvclass">)
            n257 = Format Into String(format string="Home started on wheel %d", "Wheel To Home") -> (resulting string=w484:string)  [unwired: 2 in, 1 out]
            n258 = call "CC System Message.vi"("error in (no error)"=w481, "Message"=w484) -> ("error out"=w477:errorcluster)  [unwired: 9 in]
            n259 = Get Date/Time In Seconds() -> (seconds since 1Jan1904=w467:timestamp)
            n260 = call-dynamic "Write Wheel Run State.vi"("error in (no error)"=w477, "Run"=TRUE, "Wheel"="Wheel To Home", "Filter Wheel in"=w480) -> ("error out"=w469:errorcluster, "Filter Wheel out"=w472:refnum<class "Filter Wheel.lvclass">)  [unwired: 6 in]
            n261 = Generate User Event(user event=w476, event data cluster="send data" ("event data")) -> (user event out=w475:refnum<user-event>)  [unwired: 2 in, 1 out]
            n262 = Bundle By Name(cluster=w465, "Period"=1.0, "next poll"=w467) -> (w466:T13)
            n263 = call-dynamic "Get Status.vi"("error in (no error)"=w469, "Filter Wheel in"=w472) -> ("FW Status"=w470:T11, "Filter Wheel out"=w471:refnum<class "Filter Wheel.lvclass">)  [unwired: 7 in, 1 out]
            n264 = Generate User Event(user event=w475, event data cluster="Home Finish" ("event data")) -> ()  [unwired: 2 in, 2 out]
            n265 = Bundle By Name(cluster=w466, "Filter Wheel ref"=w471, "FW Status"=w470) -> (w483:T13)
          }
          frame "Home Finish" {
            w492 = FALSE ("Visible")
            n266 = local read "Wheel To Home"() -> (w488:u16)
            n267 = Unbundle By Name(w494) -> ("Home Repeats"=w486:i32, "state"=w495:refnum<user-event>, "Filter Wheel ref"=w498:refnum<class "Filter Wheel.lvclass">)
            n268 = call-dynamic "Home Filter Wheel.vi"("Motor"=w488, "Filter Wheel in"=w498) -> ("error out"=w496:errorcluster, "Log"=w497:string, "Filter Wheel out"=w490:refnum<class "Filter Wheel.lvclass">)  [unwired: 6 in, 1 out]
            n269 = call-dynamic "Write Wheel Run State.vi"("Run"=FALSE, "Wheel"=w488, "Filter Wheel in"=w490) -> ("Filter Wheel out"=w489:refnum<class "Filter Wheel.lvclass">)  [unwired: 7 in, 1 out]
            n270 = call "CC System Message.vi"("Message"=w497) -> ("error out"=w491:errorcluster)  [unwired: 10 in]
            n271 = case shown="Error .." w496 {
              selector: w496 -> [_ w517]
              tunnel: w495 -> [w500 w515]
              tunnel: w494 -> [w504 w518]
              tunnel: [w505 w516] -> w493
              tunnel: w489 -> [w506 _]
              tunnel: w486 -> [w502 _]
              frame No Error {
                n272 = case shown="True" "Repeat Home" {
                  tunnel: w502 -> [_ w511]
                  tunnel: [0 w510] -> w501
                  tunnel: w500 -> [_ w509]
                  frame False {
                  }
                  frame True {
                    n273 = Increment(x=w511) -> (x+1=w510:i32)
                    "Repeats" <- w510
                    n274 = Generate User Event(user event=w509, event data cluster="Home" ("event data")) -> ()  [unwired: 2 in, 2 out]
                  }
                }
                n275 = Bundle By Name(cluster=w504, "Filter Wheel ref"=w506, "Period"=30.0, "Home Repeats"=w501) -> (w505:T13)
              }
              frame Error {
                n276 = Generate User Event(user event=w515, event data cluster="Error" ("event data")) -> ()  [unwired: 2 in, 2 out]
                n277 = Bundle By Name(cluster=w518, "error"=w517, "Error State"="Homing") -> (w516:T13)
                n278 = property on="Repeat Home" class="Bool (strict)"("Value"=FALSE ("Repeat Home")) -> ()  [unwired: 2 in, 2 out]
              }
            }
            n279 = property on="Moving Message" class="Str"(error in=w491, "Visible"=w492, "Blinking"=w492) -> ()  [unwired: 1 in, 2 out]
          }
          frame "Stop" {
            n280 = Unbundle By Name(w520) -> ("Filter Wheel ref"=w524:refnum<class "Filter Wheel.lvclass">)
            n281 = call-dynamic "Emergency Stop.vi"("Wheel (-1: all)"=-1, "Filter Wheel in"=w524) -> ("Filter Wheel out"=w522:refnum<class "Filter Wheel.lvclass">)  [unwired: 8 in, 1 out]
            n282 = Bundle By Name(cluster=w520, "Filter Wheel ref"=w522) -> (w521:T13)
            n283 = call "CC System Message.vi"("Message"="Filter Wheel stopped by user.") -> ()  [unwired: 10 in, 1 out]
          }
          frame "Poll" {
            # "Request status from hardware"
            n284 = Unbundle By Name(w533) -> ("state"=w532:refnum<user-event>, "Filter Wheel ref"=w527:refnum<class "Filter Wheel.lvclass">)
            n285 = property on="Filter Wheel Displays" class="Clust (strict)"() -> ("Controls[]"=w538:refnum<vi>[])  [unwired: 2 in, 2 out]
            n286 = call-dynamic "Get Status.vi"("Filter Wheel in"=w527) -> ("error out"=w529:errorcluster, "FW Status"=w526:T11, "Filter Wheel out"=w530:refnum<class "Filter Wheel.lvclass">)  [unwired: 8 in]
            n287 = call-dynamic "Read Home State.vi"("Filter Wheel in"=w527) -> ("Home State"=→"Homed":bool[])  [unwired: 8 in, 2 out]
            n288 = Generate User Event(user event=w532, event data cluster="send data" ("event data")) -> ()  [unwired: 2 in, 2 out]
            n289 = Split 1D Array(array=w538, index=8) -> (first subarray=w535:refnum<vi>[], second subarray=w536:refnum<vi>[])
            n290 = Unbundle By Name(w526) -> ("Notch"=→"On the notch":bool[])
            n291 = case shown="No Error" w529 {
              tunnel: w536 -> [w543 _]
              tunnel: w535 -> [w542 _]
              tunnel: w526 -> [w540 _]
              frame No Error {
                n292 = Unbundle By Name(w540) -> ("Positions"=w539:i32[], "Notch"=w541:bool[])
                n293 = call "Filter Wheel Update Status.vi"("FW Status"=w540) -> ()  [unwired: 10 in, 1 out]
                n294 = for {
                  tunnel: w541 -> [w545] mode=indexing
                  tunnel: w539 -> [w546] mode=indexing
                  tunnel: w543 -> [w548] mode=indexing
                  tunnel: w542 -> [w547] mode=indexing
                  n295 = Not(x=w545) -> ()  [unwired: 1 out]
                  n296 = property class="Ctl"(reference=w548, "Value"=w546) -> ()  [unwired: 1 in, 2 out]
                  n297 = property class="Ctl"(reference=w547, "Blinking"=FALSE, "Value"=w546) -> ()  [unwired: 1 in, 2 out]
                }
              }
              frame Error {
              }
            }
            n298 = Bundle By Name(cluster=w533, "Filter Wheel ref"=w530, "FW Status"=w526) -> (w534:T13)
          }
          frame "send raw string" {
            n299 = Unbundle By Name(w549) -> ("Filter Wheel ref"=w553:refnum<class "Filter Wheel.lvclass">)
            n300 = call-dynamic "Send Raw String.vi"("Cmd String"="Command Preview", "Filter Wheel in"=w553) -> ("Filter Wheel out"=w551:refnum<class "Filter Wheel.lvclass">)  [unwired: 8 in, 1 out]
            n301 = Bundle By Name(cluster=w549, "Filter Wheel ref"=w551) -> (w550:T13)
          }
          frame "read raw" {
            n302 = Unbundle By Name(w557) -> ("Filter Wheel ref"=w556:refnum<class "Filter Wheel.lvclass">)
            n303 = call-dynamic "Read Raw String.vi"("Filter Wheel in"=w556) -> ("Raw String"=→"Response":string, "Filter Wheel out"=w555:refnum<class "Filter Wheel.lvclass">)  [unwired: 8 in, 1 out]
            n304 = Bundle By Name(cluster=w557, "Filter Wheel ref"=w555) -> (w558:T13)
          }
          frame "Send Config" {
            n305 = Unbundle By Name(w564) -> ("Data Q"=w563:refnum<queue>, "Filter Wheel Info"=w560:T7)
            n306 = Bundle By Name(cluster=T16 {"Source"="", "Type"="", "Data"=variant} ("element"), "Source"="Filter Wheel Config" ("Data Type"), "Data"=w560) -> (w559:T16)
            n307 = Enqueue Element(queue=w563, element=w559) -> ()  [unwired: 2 in, 3 out]
          }
          frame "Send Status" {
            n308 = Unbundle By Name(w571) -> ("Data Q"=w570:refnum<queue>, "Filter Wheel ref"=w566:refnum<class "Filter Wheel.lvclass">)
            n309 = call-dynamic "Get Status.vi"("Filter Wheel in"=w566) -> ("FW Status"=w565:T11)  [unwired: 8 in, 2 out]
            n310 = Bundle By Name(cluster=T16 {"Source"="", "Type"="", "Data"=variant} ("element"), "Source"="Filter Wheel Status" ("Data Type"), "Data"=w565) -> (w567:T16)
            n311 = Enqueue Element(queue=w570, element=w567) -> ()  [unwired: 2 in, 3 out]
          }
          frame "Error" {
            w578 = "Filter Wheel" ("Source")
            n312 = Unbundle By Name(w576) -> ("error.status"=w585:bool, "Data Q"=w581:refnum<queue>, "Error State"=w573:string)
            n313 = Bundle By Name(cluster=T20 {"Measured Value"=0.0, "Alarm Low"=0.0, "Alarm High"=0.0, "Message"="", "Source"=""} ("element"), "Source"=w578, "Message"=w573) -> (w579:T20)
            n314 = property on="Error" class="Bool (strict)"("Value"=w585) -> ()  [unwired: 2 in, 2 out]
            n315 = Bundle By Name(cluster=T16 {"Source"="", "Type"="", "Data"=variant} ("element"), "Source"=w578, "Type"="Alarm Set", "Data"=w579) -> (w582:T16)
            n316 = Format Into String(format string="Filter Wheel Error: %s", w573) -> (resulting string=w572:string)  [unwired: 2 in, 1 out]
            n317 = Enqueue Element(queue=w581, element=w582) -> ()  [unwired: 2 in, 3 out]
            n318 = Bundle By Name(cluster=w576, "Period"=30.0) -> (w577:T13)
            n319 = call "CC System Message.vi"("Message"=w572) -> ()  [unwired: 10 in, 1 out]
          }
          frame "Ready" {
            w589 = "Filter Wheel" ("Source")
            n320 = Unbundle By Name(w597) -> ("Data Q"=w593:refnum<queue>, "Error State"=w590:string)
            n321 = Bundle By Name(cluster=T20 {"Measured Value"=0.0, "Alarm Low"=0.0, "Alarm High"=0.0, "Message"="", "Source"=""} ("element"), "Source"=w589, "Message"=w590) -> (w591:T20)
            n322 = Bundle By Name(cluster=T16 {"Source"="", "Type"="", "Data"=variant} ("element"), "Source"=w589, "Type"="Alarm Clear", "Data"=w591) -> (w594:T16)
            n323 = Enqueue Element(queue=w593, element=w594) -> (error out=w587:errorcluster)  [unwired: 2 in, 2 out]
            n324 = call "CC System Message.vi"("Message"="Filter Wheel Ready") -> ()  [unwired: 10 in, 1 out]
            n325 = property on="Error" class="Bool (strict)"(error in=w587, "Value"=FALSE ("Error")) -> ()  [unwired: 1 in, 2 out]
          }
          frame "Shutdown" {
            n326 = Unbundle By Name(w600) -> ("Filter Wheel ref"=w599:refnum<class "Filter Wheel.lvclass">)
            n327 = call-dynamic "Close.vi"("Filter Wheel in"=w599) -> ()  [unwired: 9 in, 2 out]
            n328 = call "CC System Message.vi"("Message"="Filter Wheel shutdown.") -> ()  [unwired: 10 in, 1 out]
          }
        }
      }
      event "Wheel To Home": Value Change {
        n329 = event-data() -> ("NewVal"=w607:u16)  [unwired: 1 in]
        n330 = Not Equal?(x=w607, y=u16 3) -> (x != y?=w605:bool)
        n331 = Select(t=T21."Enabled" ("Disabled"), s=w605, f=T21."Disabled and Grayed Out" ("Disabled")) -> (s? t:f=w602:T21)
        n332 = property on="Home" class="Bool"("DisabledEnum"=w602) -> ()  [unwired: 2 in, 2 out]
      }
      event "Save Slit Wheel Pos": Value Change {
        n333 = event-data() -> ()  [unwired: 1 in, 6 out]
        n334 = Unbundle By Name(w614) -> ("Filter Wheel ref"=w617:refnum<class "Filter Wheel.lvclass">)
        n335 = call "Update Position.vi"("Position (0:4)"="Slit Wheel Location", "Filter Wheel (0:n-1)"=3, "Filter Wheel in"=w617) -> ("Filter Wheel out"=w609:refnum<class "Filter Wheel.lvclass">)  [unwired: 7 in, 1 out]
        n336 = To More Specific Class(target class=refnum<class "FW Arduino Control.lvclass"> refnum ("FW Arduino Control.lvclass"), reference=w609) -> (specific class reference=w611:refnum<class "FW Arduino Control.lvclass">)  [unwired: 1 in, 1 out]
        n337 = call "FW Arduino Rd Wr Settings.vi"("Write? (F:Read)"=TRUE, "Settings"=w611) -> ()  [unwired: 8 in, 2 out]
        n338 = Bundle By Name(cluster=w614, "Filter Wheel ref"=w609) -> (w613:T13)
      }
      event "Positions": Shortcut Menu Activation? {
        n339 = event-data() -> ("CtlRef"=w623:refnum<vi>, "Coords"=w622:T22)  [unwired: 1 in, 5 out]
        n340 = invoke class="MCListbox (strict)" method="Point To Row Column"(reference=w623, "Point"=w622) -> ("CellPosition"=w620:T10)  [unwired: 5 in, 6 out]
        n341 = Bundle By Name(cluster=w618, "Coords"=w620) -> (w619:T13)
        n342 = event-data("Discard?"=FALSE) -> ()  [unwired: 1 in, 1 out]
      }
      event "Positions": Shortcut Menu Selection (User) {
        n343 = event-data() -> ()  [unwired: 1 in, 8 out]
        n344 = Unbundle By Name(w624) -> ("Pos Names"=w634:cluster{"Table":string[][]}[], "Coords.Row"=w628:i32)
        n345 = local read "Wheels"() -> (w631:i32)
        n346 = Index Array(array=w634, index=w631) -> (element=w635:cluster{"Table":string[][]})
        n347 = Unbundle(w635) -> ("Table"=w630:string[][])
        n348 = Array Size(array=w630) -> (size(s)=w629:i32[])
        n349 = Index Array(array=w629) -> (element=w627:i32)  [unwired: 1 in]
        n350 = for {
          N: w627 -> [_]
          tunnel: w630 -> [w642]
          tunnel: w628 -> [w640]
          tunnel: w627 -> [w637]
          tunnel: [w636] -> w626 mode=indexing
          i -> [w641]
          n351 = Add(x=w640, y=w641) -> (x+y=w638:i32)
          n352 = Quotient & Remainder(x=w638, y=w637) -> (x-y*floor(x/y)=w639:i32)  [unwired: 1 out]
          n353 = Index Array(array=w642, index (row)=w639) -> (element=w636:string[])  [unwired: 1 in]
        }
        n354 = Bundle("Table"=w626) -> (w633:cluster{"Table":string[][]})  [unwired: 1 in]
        n355 = Replace Array Subset(array=w634, new element=w633, index=w631) -> (w632:cluster{"Table":string[][]}[])
        n356 = Bundle By Name(cluster=w624, "Pos Names"=w632) -> (w625:T13)
        n357 = property on="Positions" class="MCListbox (strict)"("ItemNames"=w626) -> ()  [unwired: 2 in, 2 out]
      }
      event "Standalone": Value Change {
        n358 = event-data() -> ("NewVal"=w643:bool)  [unwired: 1 in]
        n359 = property on="Close" class="Bool"("Visible"=w643) -> ()  [unwired: 2 in, 2 out]
      }
      event "Alarms?": Value Change {
        n360 = event-data() -> ()  [unwired: 1 in, 6 out]
        n361 = Unbundle By Name(w646) -> ("Filter Wheel ref"=w649:refnum<class "Filter Wheel.lvclass">)
        n362 = property class="Filter Wheel.lvclass"(reference=w649, "Alarms_"="Alarms?") -> (reference out=w647:refnum<class "Filter Wheel.lvclass">)  [unwired: 1 in, 1 out]
        n363 = Bundle By Name(cluster=w646, "Filter Wheel ref"=w647) -> (w645:T13)
      }
      event "Open Arduino Log": Value Change {
        n364 = event-data() -> ()  [unwired: 1 in, 6 out]
        n365 = Unbundle By Name(w655) -> ()  [unwired: 1 out]
        n366 = call <vilib>:"Dflt Data Dir.vi"() -> ("App:Default Data Directory"=w654:path)
        n367 = Build Path(base path=w654, name or relative path="Logs") -> (appended path=w652:path)
        n368 = Build Path(base path=w652, name or relative path="Filter Wheel") -> (appended path=w650:path)
        n369 = call <vilib>:"Show in File System.vi"("file or directory path"=w650) -> ()  [unwired: 10 in, 1 out]
      }
      event "Read": Value Change {
        n370 = event-data() -> ()  [unwired: 1 in, 6 out]
        n371 = Unbundle By Name(w658) -> ("state"=w657:refnum<user-event>)
        n372 = Generate User Event(user event=w657, event data cluster="read raw" ("event data")) -> ()  [unwired: 2 in, 2 out]
      }
      event "Error": Value Change {
        n373 = event-data() -> ()  [unwired: 1 in, 6 out]
        n374 = Unbundle By Name(w660) -> ("Error State"=w661:string, "error.code"=w668:i32, "error.source"=w667:string, "error.status"=w666:bool)
        n375 = Format Into String(format string="An error occurred during %s. \nError Number: %d\nError message: %s", w661, w668, w667) -> (resulting string=w665:string)  [unwired: 2 in, 1 out]
        n376 = call "Display Message to User"("Enable"=w666, "Message"=w665) -> ("error out"=w662:errorcluster, "Close"=w664:bool)  [unwired: 8 in]
        n377 = Unbundle By Name(w660) -> ("state"=w659:refnum<user-event>)
        n378 = case shown="True" w664 {
          selector: w664 -> [w670 _]
          tunnel: w660 -> [w673 w676]
          tunnel: [w671 w676] -> w663
          tunnel: w662 -> [w672 _]
          tunnel: w659 -> [_ w675]
          frame False {
            n379 = property on="Error" class="Bool (strict)"("Value"=w670) -> ()  [unwired: 2 in, 2 out]
            n380 = Bundle By Name(cluster=w673, "error"=w672) -> (w671:T13)
          }
          frame True {
            n381 = Generate User Event(user event=w675, event data cluster="Ready" ("event data")) -> ()  [unwired: 2 in, 2 out]
          }
        }
      }
      event "Homing": Value Change {
        n382 = event-data() -> ()  [unwired: 1 in, 6 out]
        n383 = Unbundle By Name(w682) -> ("Filter Wheel ref"=w685:refnum<class "Filter Wheel.lvclass">, "Name"=w680:string)
        n384 = call-dynamic "Write Homing.vi"("Homing"="Homing", "Filter Wheel in"=w685) -> ("Filter Wheel out"=w684:refnum<class "Filter Wheel.lvclass">)  [unwired: 8 in, 1 out]
        n385 = Bundle By Name(cluster=w682, "Filter Wheel ref"=w684) -> (w683:T13)
        n386 = call "Rd Wr Filter Wheel Settings.vi"("Wheel Name"=w680) -> ("Filter Wheel Settings"=w679:T7)  [unwired: 9 in, 1 out]
        n387 = Bundle By Name(cluster=w679, "Homing"="Homing") -> (w678:T7)
        n388 = call "Rd Wr Filter Wheel Settings.vi"("Wheel Name"=w680, "Write? (F:Read)"=TRUE, "Filter Wheel Info"=w678) -> ()  [unwired: 7 in, 2 out]
      }
      event "Default Speed": Value Change {
        n389 = event-data() -> ()  [unwired: 1 in, 6 out]
        n390 = Unbundle By Name(w689) -> ("Filter Wheel ref"=w695:refnum<class "Filter Wheel.lvclass">, "Name"=w686:string)
        n391 = call-dynamic "Read Filter Wheel Info.vi"("Filter Wheel in"=w695) -> ("Filter Wheel Info"=w693:T7, "Filter Wheel out"=w694:refnum<class "Filter Wheel.lvclass">)  [unwired: 8 in, 1 out]
        n392 = Bundle By Name(cluster=w693, "Default Speed"="Default Speed") -> (w687:T7)
        n393 = call-dynamic "Write Filter Wheel Info.vi"("Filter Wheel Info"=w687, "Filter Wheel in"=w694) -> ("Filter Wheel out"=w691:refnum<class "Filter Wheel.lvclass">)  [unwired: 8 in, 1 out]
        n394 = call "Rd Wr Filter Wheel Settings.vi"("Wheel Name"=w686, "Write? (F:Read)"=TRUE, "Filter Wheel Info"=w687) -> ()  [unwired: 7 in, 2 out]
        n395 = Bundle By Name(cluster=w689, "Filter Wheel ref"=w691) -> (w690:T13)
      }
      event "Home": Value Change {
        n396 = event-data() -> ()  [unwired: 1 in, 6 out]
        n397 = Unbundle By Name(w698) -> ("state"=w697:refnum<user-event>)
        n398 = Generate User Event(user event=w697, event data cluster="Home" ("event data")) -> ()  [unwired: 2 in, 2 out]
      }
      event "Repeat Home": Value Change {
        n399 = event-data() -> ()  [unwired: 1 in, 6 out]
        n400 = Unbundle By Name(w701) -> ("state"=w703:refnum<user-event>)
        n401 = Generate User Event(user event=w703, event data cluster="Home" ("event data")) -> ()  [unwired: 2 in, 2 out]
        n402 = local write "Wheel To Home"("Wheel ID") -> ()
        n403 = property on="Repeats" class="DigNum (strict)"("Value"=0 ("Repeats")) -> ()  [unwired: 2 in, 2 out]
      }
      event "Simulate": Value Change {
        n404 = event-data() -> ()  [unwired: 1 in, 6 out]
        n405 = Unbundle By Name(w709) -> ("state"=w708:refnum<user-event>)
        n406 = Select(t="set simulation on" ("event data"), s="Simulate", f="set simulation off" ("event data")) -> (s? t:f=w705:string)
        n407 = Generate User Event(user event=w708, event data cluster=w705) -> ()  [unwired: 2 in, 2 out]
      }
      event "Sim Velocity (steps/sec)": Value Change {
        n408 = event-data() -> ()  [unwired: 1 in, 6 out]
        n409 = Unbundle By Name(w710) -> ("Simulate"=w713:bool, "Filter Wheel ref"=w714:refnum<class "Filter Wheel.lvclass">)
        n410 = case shown="True" w713 {
          tunnel: w714 -> [_ w722]
          tunnel: "Sim Velocity (steps/sec)" -> [_ w719]
          tunnel: w710 -> [w715 w718]
          tunnel: [w715 w716] -> w711
          frame False {
          }
          frame True {
            n411 = To More Specific Class(target class=refnum<class "Filter Wheel Simulator.lvclass"> refnum ("Filter Wheel Simulator.lvclass"), reference=w722) -> (specific class reference=w720:refnum<class "Filter Wheel Simulator.lvclass">)  [unwired: 1 in, 1 out]
            n412 = call "Write Velocity (cnts_sec).vi"("Velocity (cnts/sec)"=w719, "Filter Wheel Simulator in"=w720) -> ("Filter Wheel Simulator out"=w717:refnum<class "Filter Wheel Simulator.lvclass">)  [unwired: 8 in, 1 out]
            n413 = Bundle By Name(cluster=w718, "Filter Wheel ref"=w717) -> (w716:T13)
          }
        }
      }
      event "Connect": Value Change {
        n414 = event-data() -> ()  [unwired: 1 in, 6 out]
        n415 = Unbundle By Name(w725) -> ("state"=w724:refnum<user-event>)
        n416 = Generate User Event(user event=w724, event data cluster="connect" ("event data")) -> ()  [unwired: 2 in, 2 out]
      }
      event Value Change {
        n417 = event-data() -> ()  [unwired: 1 in, 1 out]
        n418 = Unbundle By Name(w728) -> ("state"=w727:refnum<user-event>)
        n419 = Generate User Event(user event=w727, event data cluster="show command" ("event data")) -> ()  [unwired: 2 in, 2 out]
      }
      event "Send Command": Value Change {
        n420 = event-data() -> ()  [unwired: 1 in, 6 out]
        n421 = Unbundle By Name(w731) -> ("state"=w730:refnum<user-event>)
        n422 = Generate User Event(user event=w730, event data cluster="send raw string" ("event data")) -> ()  [unwired: 2 in, 2 out]
      }
      event "STOP": Value Change {
        n423 = event-data() -> ()  [unwired: 1 in, 6 out]
        n424 = Unbundle By Name(w734) -> ("state"=w733:refnum<user-event>)
        n425 = Generate User Event(user event=w733, event data cluster="Stop" ("event data")) -> ()  [unwired: 2 in, 2 out]
      }
      event Value Change {
        n426 = event-data() -> ()  [unwired: 1 in, 1 out]
        n427 = Unbundle By Name(w737) -> ("state"=w736:refnum<user-event>)
        n428 = Generate User Event(user event=w736, event data cluster="set mode" ("event data")) -> ()  [unwired: 2 in, 2 out]
      }
      event "Filter Wheel Displays": Value Change {
        n429 = event-data() -> ("OldVal"=w745:T3, "NewVal"=w738:T3)  [unwired: 1 in]
        n430 = Unbundle By Name(w746) -> ("state"=w749:refnum<user-event>)
        n431 = Not Equal?(x=w745, y=w738) -> (x != y?=w744:T23)
        n432 = Cluster To Array(cluster=w738) -> (array=w741:i32[])
        n433 = Cluster To Array(cluster=w744) -> (array=w743:bool[])
        n434 = Generate User Event(user event=w749, event data cluster="Move" ("event data")) -> ()  [unwired: 2 in, 2 out]
        n435 = Search 1D Array(1D array=w743, element=TRUE) -> (index of element=w739:i32)  [unwired: 1 in]
        n436 = Index Array(array=w741, index=w739) -> (element=w740:i32)
        n437 = Bundle By Name(cluster=w746, "Move.Wheel ID"=w739, "Move.Position"=w740) -> (w747:T13)
      }
      event "Wheels": Value Change {
        n438 = event-data() -> ("NewVal"=w752:i32)  [unwired: 1 in]
        n439 = Unbundle By Name(w750) -> ("Pos Names"=w755:cluster{"Table":string[][]}[])
        n440 = Index Array(array=w755, index=w752) -> (element=w754:cluster{"Table":string[][]})
        n441 = Unbundle(w754) -> ("Table"=w753:string[][])
        n442 = property on="Positions" class="MCListbox (strict)"("ItemNames"=w753) -> ()  [unwired: 2 in, 2 out]
        n443 = Bundle By Name(cluster=w750, "Wheel"=w752) -> (w751:T13)
      }
      event "Wheels": Edit Cell? {
        n444 = event-data() -> ("String"=w760:string, "Coords"=w759:T10)  [unwired: 1 in]
        n445 = Unbundle By Name(w759) -> ("Column"=w762:i32)
        n446 = Equal?(x=1, y=w762) -> (x = y?=w761:bool)
        n447 = Bundle By Name(cluster=w757, "Coords"=w759) -> (w758:T13)
        n448 = event-data("String"=w760, "Discard?"=w761) -> ()  [unwired: 1 in, 1 out]
      }
      event "Wheels": Edit Cell {
        n449 = event-data() -> ("String"=w769:string)  [unwired: 1 in]
        n450 = Unbundle By Name(w767) -> ("Filter Wheel Info.Filters"=w764:T8[], "FW names"=w770:string[], "Coords.Row"=w766:i32, "Coords.Column"=w765:i32, "state"=w763:refnum<user-event>)
        n451 = case shown="0, Default" w765 {
          tunnel: w770 -> [w776 _ _]
          tunnel: w769 -> [w775 _ w787]
          tunnel: [w773 w777 w780] -> w768
          tunnel: w767 -> [w772 w777 w782]
          tunnel: w766 -> [w771 _ w784]
          tunnel: w764 -> [_ _ w785]
          tunnel: w763 -> [_ _ w779]
          frame 0, Default {
            n452 = Replace Array Subset(array=w776, new element=w775, index=w771) -> (w774:string[])
            n453 = Bundle By Name(cluster=w772, "FW names"=w774) -> (w773:T13)
          }
          frame 1 {
          }
          frame 2 {
            n454 = Decimal String To Number(string=w787) -> (number=w786:i32)  [unwired: 2 in, 1 out]
            n455 = Index Array(array=w785, index=w784) -> (element=w788:T8)
            n456 = Generate User Event(user event=w779, event data cluster="Show Filter Wheels" ("event data")) -> ()  [unwired: 2 in, 2 out]
            n457 = Bundle By Name(cluster=w788, "Size"=w786) -> (w783:T8)
            n458 = Replace Array Subset(array=w785, new element=w783, index=w784) -> (w781:T8[])
            n459 = Bundle By Name(cluster=w782, "Filter Wheel Info.Filters"=w781) -> (w780:T13)
          }
        }
      }
      event "Positions": Edit Cell? {
        n460 = event-data() -> ("String"=w794:string, "Coords"=w791:T10)  [unwired: 1 in, 4 out]
        n461 = Unbundle By Name(w791) -> ("Column"=w795:i32)
        n462 = case shown="1" w795 {
          tunnel: w794 -> [w797 w803]
          tunnel: [w797 w800] -> w793
          tunnel: [FALSE ("status") w798] -> w792
          frame 0, Default {
          }
          frame 1 {
            w802 = "%d" ("format string")
            n463 = Scan From String(format string=w802, input string=w803) -> (error out=w799:errorcluster, output 1=w801:i32)  [unwired: 3 in, 2 out]
            n464 = Unbundle By Name(w799) -> ("status"=w798:bool)
            n465 = Format Into String(format string=w802, w801) -> (resulting string=w800:string)  [unwired: 2 in, 1 out]
          }
        }
        n466 = Bundle By Name(cluster=w789, "Coords"=w791) -> (w790:T13)
        n467 = event-data("String"=w793, "Discard?"=w792) -> ()  [unwired: 1 in, 1 out]
      }
      event "Positions": Edit Cell {
        n468 = event-data() -> ("String"=w812:string)  [unwired: 1 in, 5 out]
        n469 = Unbundle By Name(w805) -> ("Pos Names"=w810:cluster{"Table":string[][]}[], "Coords"=w804:T10)
        n470 = Unbundle By Name(w804) -> ("Row"=w813:i32, "Column"=w814:i32)
        n471 = Index Array(array=w810, index="Wheels") -> (element=w816:cluster{"Table":string[][]})
        n472 = Unbundle(w816) -> ("Table"=w815:string[][])
        n473 = Replace Array Subset(array=w815, new element=w812, index (row)=w813, index (col)=w814) -> (w811:string[][])
        n474 = Bundle("Table"=w811) -> (w809:cluster{"Table":string[][]})  [unwired: 1 in]
        n475 = Replace Array Subset(array=w810, new element=w809, index="Wheels") -> (w807:cluster{"Table":string[][]}[])
        n476 = Bundle By Name(cluster=w805, "Pos Names"=w807) -> (w806:T13)
      }
      event "Add Pos": Value Change {
        n477 = event-data() -> ()  [unwired: 1 in, 6 out]
        n478 = Unbundle By Name(w827) -> ("Pos Names"=w823:cluster{"Table":string[][]}[], "Wheel"=w822:i32)  [unwired: 1 out]
        n479 = Index Array(array=w823, index=w822) -> (element=w821:cluster{"Table":string[][]})
        n480 = Build Array("Unnamed", "0") -> (w824:string[])
        n481 = Unbundle By Name(w821) -> ("Table"=w818:string[][])
        n482 = Build Array (concatenate)(w818, w824) -> (w817:string[][])
        n483 = Bundle By Name(cluster=w821, "Table"=w817) -> (w820:cluster{"Table":string[][]})
        n484 = property on="Positions" class="MCListbox (strict)"("ItemNames"=w817) -> ()  [unwired: 2 in, 2 out]
        n485 = Replace Array Subset(array=w823, new element=w820, index=w822) -> (w819:cluster{"Table":string[][]}[])
        n486 = Bundle By Name(cluster=w827, "Pos Names"=w819) -> (w828:T13)
      }
      event "Remove Pos": Value Change {
        n487 = event-data() -> ()  [unwired: 1 in, 6 out]
        n488 = Unbundle By Name(w836) -> ("Pos Names"=w830:cluster{"Table":string[][]}[], "Wheel"=w835:i32)
        n489 = Index Array(array=w830, index=w835) -> (element=w832:cluster{"Table":string[][]})
        n490 = Unbundle By Name(w832) -> ("Table"=w834:string[][])
        n491 = Delete From Array(array=w834, index (row)="Positions") -> (array with subset deleted=w829:string[][])  [unwired: 2 in, 1 out]
        n492 = Bundle By Name(cluster=w832, "Table"=w829) -> (w831:cluster{"Table":string[][]})
        n493 = property on="Positions" class="MCListbox (strict)"("ItemNames"=w829) -> ()  [unwired: 2 in, 2 out]
        n494 = Replace Array Subset(array=w830, new element=w831, index=w835) -> (w838:cluster{"Table":string[][]}[])
        n495 = Bundle By Name(cluster=w836, "Pos Names"=w838) -> (w837:T13)
      }
      event "Add Fw": Value Change {
        n496 = event-data() -> ()  [unwired: 1 in, 6 out]
        n497 = Unbundle By Name(w842) -> ("FW names"=w840:string[], "Pos Names"=w841:cluster{"Table":string[][]}[])
        n498 = Array Size(array=w840) -> (size(s)=w839:i32)
        n499 = case shown="0..4" w839 {
          tunnel: w840 -> [_ w861]
          tunnel: [w845 w860] -> w843
          tunnel: w842 -> [w845 w859]
          tunnel: w841 -> [_ w848]
          frame 5, Default {
            n500 = One Button Dialog(message="Maximum of 4 filter wheels") -> ()  [unwired: 1 in, 1 out]
          }
          frame 0..4 {
            w852 = "Unnamed"
            n501 = Build Array (concatenate)(w848, cluster{"Table":string[][]} {"Table"=[]}) -> (w846:cluster{"Table":string[][]}[])
            n502 = property on="Wheels" class="MCListbox (strict)"() -> ("ItemNames"=w853:string[][])  [unwired: 2 in, 2 out]
            n503 = Build Array (concatenate)(w861, w852) -> (w855:string[])
            n504 = Build Array(w852, "0" ("element")) -> (w850:string[])
            n505 = Array Size(array=w855) -> (size(s)=w857:i32)
            n506 = Decrement(x=w857) -> (x-1=w856:i32)
            n507 = Build Array (concatenate)(w853, w850) -> (w849:string[][])
            n508 = property on="Wheels" class="MCListbox (strict)"("ItemNames"=w849) -> (error out=w854:errorcluster)  [unwired: 2 in, 1 out]
            n509 = Bundle By Name(cluster=T10 {"Row"=0, "Column"=0} ("Active Cell:Active Cell"), "Row"=w856) -> (w858:T10)
            n510 = Bundle By Name(cluster=w859, "Filter Wheel Info.Num Wheels"=w857, "FW names"=w855, "Pos Names"=w846) -> (w860:T13)
            n511 = property on="Wheels" class="MCListbox (strict)"(error in=w854, "ActiveCell"=w858, "FocusRow"=w856) -> ()  [unwired: 1 in, 2 out]
          }
        }
      }
      event "Remove Fw": Value Change {
        w867 = 1 ("length")
        n512 = event-data() -> ()  [unwired: 1 in, 6 out]
        n513 = Unbundle By Name(w865) -> ("FW names"=w872:string[], "Pos Names"=w871:cluster{"Table":string[][]}[], "Wheel"=w870:i32, "state"=w864:refnum<user-event>)
        n514 = Generate User Event(user event=w864, event data cluster="Show Tables" ("event data")) -> ()  [unwired: 2 in, 2 out]
        n515 = Delete From Array(array=w872, length=w867, index=w870) -> (array with subset deleted=w869:string[])  [unwired: 1 out]
        n516 = Delete From Array(array=w871, length=w867, index=w870) -> (array with subset deleted=w868:cluster{"Table":string[][]}[])  [unwired: 1 out]
        n517 = Bundle By Name(cluster=w865, "FW names"=w869, "Pos Names"=w868) -> (w866:T13)
      }
      event "Save Button": Value Change {
        # "\"Filter Wheel Settings Simulation\":{\n    \"Addr\":\"\",\n    \"Filters\":[\n      {\n        \"Names\":[\"Y\",\"J\",\"H\",\"Open\"],\n        \"Relative Position\":[1,2,3,4],\n        \"Wheel Name\":\"YJH\"\n      },\n      {\n        \"Names\":[\"Z\",\"Narrow\",\"Dark\",\"Open\"],\n        \"Relative Position\":[1,2,3,4],\n        \"Wheel Name\":\"NarrowBand\"\n      }"
        # "Need to copy data from array to filter wheel info cluster"
        n518 = event-data() -> ()  [unwired: 1 in, 6 out]
        n519 = Unbundle By Name(w878) -> ("state"=w876:refnum<user-event>, "Filter Wheel ref"=w885:refnum<class "Filter Wheel.lvclass">, "Filter Wheel Info"=w874:T7, "FW names"=w884:string[], "Pos Names"=w883:cluster{"Table":string[][]}[])
        n520 = Unbundle By Name(w874) -> ("Filters"=w873:T8[])
        n521 = for {
          tunnel: w884 -> [w897] mode=indexing
          tunnel: w883 -> [w896] mode=indexing
          tunnel: [w889] -> w881 mode=indexing
          tunnel: w873 -> [w888]
          i -> [w887]
          n522 = Unbundle(w896) -> ("Table"=w893:string[][])
          n523 = Index Array(array=w893, index (col)=0 ("disabled index (col)")) -> (element=w894:string[])  [unwired: 1 in]
          n524 = Index Array(array=w893, index (col)=1 ("disabled index (col)")) -> (element=w891:string[])  [unwired: 1 in]
          n525 = Decimal String To Number(string=w891) -> (number=w890:i32[])  [unwired: 2 in, 1 out]
          n526 = Index Array(array=w888, index=w887) -> (element=w886:T8)
          n527 = Bundle By Name(cluster=w886, "Wheel Name"=w897, "Relative Position"=w890, "Names"=w894) -> (w889:T8)
        }
        n528 = Generate User Event(user event=w876, event data cluster="Show Filter Wheels" ("event data")) -> ()  [unwired: 2 in, 2 out]
        n529 = Array Size(array=w881) -> (size(s)=w882:i32)
        n530 = Bundle By Name(cluster=w874, "Num Wheels"=w882, "Filters"=w881) -> (w880:T7)
        n531 = call-dynamic "Write Filter Wheel Info.vi"("Filter Wheel Info"=w880, "Filter Wheel in"=w885) -> ("Filter Wheel out"=w875:refnum<class "Filter Wheel.lvclass">)  [unwired: 8 in, 1 out]
        n532 = Bundle By Name(cluster=w878, "Filter Wheel Info"=w880, "Filter Wheel ref"=w875) -> (w879:T13)
      }
      event "Restore Defaults": Value Change {
        n533 = event-data() -> ()  [unwired: 1 in, 6 out]
        n534 = Unbundle By Name(w899) -> ("state"=w898:refnum<user-event>)
        n535 = Generate User Event(user event=w898, event data cluster="init Create Wheel" ("event data")) -> ()  [unwired: 2 in, 2 out]
      }
      event "Close": Value Change {
        n536 = event-data() -> ()  [unwired: 1 in, 2 out]
        n537 = Unbundle By Name(w903) -> ("state"=w902:refnum<user-event>)
        n538 = Generate User Event(user event=w902, event data cluster="Shutdown" ("event data")) -> ()  [unwired: 2 in, 2 out]
      }
    }
  }
  "Wheel Name" <- "Filter Wheel name"
